vi "main_monitor_Rev_17x.vi"() -> ()   [LabVIEW 2012]
uses:
  <vilib>/measure/mamon.llb/Trigger Detection for 1 Channel.vi
  <vilib>/Analysis/3filter.llb/Butterworth Filter (DBL).vi
  <vilib>/measure/matone.llb/Extract Single Tone Information 1 Chan.vi
  <vilib>/measure/NI_MAPro.lvlib
  <vilib>/Analysis/NI_AALBase.lvlib
panel:
  out "# of bytes written":dbl
  out "String":string
  out "Array":dbl[](array[numeric])
  out "Delay":u32
  in  "SHIFT INPUT1 L SEL":bool
  in  "SHIFT INPUT2 R SEL":bool
  out "INPU1 shift sign":dbl
  out "INPUT2 shift sign":dbl
  out "Message":string
  out "Message 2":string
  out "Loop Count":i32
  out "Sent Command":string
  out "Shift INPUT2 R":dbl
  out "Shift INPUT1 L":dbl
  in  "Input buffer size 2":u32=16384
  out "Connected to Name":string
  out "Range Sel IN1 in":dbl format="%.2f"
  out "Range Sel IN2 in":dbl format="%.2f"
  out "Divider INPUT1 L":dbl
  out "Divider INPUT2 R":dbl
  out "Available COM ports":string[](array[string])
  out "Current time 2":timestamp
  out "#of sent bytes":dbl
  out "Lower Loc":dbl
  out "Upper Loc":dbl
  out "Running":bool
  out "Number of Samples":dbl
  out "Bytes at Port":u32
  out "Actual bytes read":u32
  in  "Input buffer size":u32=16384
  in  "baud rate":u32=1200000
  out "RESET USB":bool
  out "Connected to:":string
  in  "Select COM port":refnum<visa-resource-name>="COM3"
  in  "CNK":T1(tab)
  in  "Send New Configuration":bool
  in  "A/D settings":u16(ring)=1 items=["Set AD to 57 ksps", "Set AD to 3.56 ksps"]
  out "OL IN2":bool
  out "OL IN1":bool
  in  "Range select INPUT2":u16(ring) items=["+/- 0.6V", "+/- 18V", "+/- 110V", "+/- 450V"]
  in  "Range select INPUT1":u16(ring) items=["+/- 0.6V", "+/- 18V", "+/- 110V", "+/- 450V"]
  in  "AC /DC INPUT 2":bool
  in  "AC/DC INPUT 1":bool
  in  "View Select":T2(tab)
  out "Voltage":dynamicdata(graph)
  in  "Async send character":bool
  in  "Refresh Delay":dbl(knob)=46.47820132563531 scale=10.0..250.0
  out "Saved Value 2 IN1":dbl
  in  "Store Value 2 IN1":bool
  out "VDC INPUT1":dbl
  out "Number of data points":dbl
  out "Waveform Graph 2":dynamicdata(graph)
  out "Saved Value 1 IN1":dbl
  in  "Store Value 1 IN1":bool
  out "VDC INPUT2":dbl format="%#.6g"
  out "INPUT1 VAC Hz":dbl format="%#.6g"
  out "INPUT2 VAC Hz":dbl format="%#.6g"
  out "VMIN IN1":dbl format="%#.5g"
  out "VMAX CH1":dbl format="%#.5g"
  out "VMIN CH1":dbl format="%#.5g"
  out "VMAX IN1":dbl format="%#.5g"
  out "VRMS INPUT2":dbl format="%#.6g"
  out "VRMS INPUT1":dbl format="%#.6g"
  out "IN1 - IN2 V shift":dbl
  out "IN1/IN2 V gain":dbl
  in  "Store Value 1 IN2":bool
  out "Saved Value 1 IN2":dbl
  out "Saved Value 2 IN2":dbl
  in  "Store Value 2 IN2":bool
  in  "INPUT 2R Loc":dbl step=0.001
  in  "INPUT 1L Loc":dbl step=0.001
  in  "Zoom In Graph --->":dbl(slide)=0.573803 min=0.0 max=0.65 step=0.001 scale format="%#_1g"
  in  "Char to send":string="6"
  out "FFT":dynamicdata(graph)
  in  "Zoom In Graph ---> 2":dbl(slide)=1000.0 min=0.0 max=0.65 step=0.001 scale format="%#_1g"
  in  "Play Button":bool
  in  "Zoom In Graph ---> 3":dbl(slide)=0.573803 min=0.0 max=0.65 step=0.001 scale format="%#_1g"
  in  "Record single value":bool
  in  "Select path and filename":path
  in  "Continuous Rec Data CH0":bool
  out "Recorded data":waveform(dbl)[](graph)
  in  "Stop Playing":bool
  in  "Play Speed":i32(knob)=1000 scale=100.0..2000.0
  out "Reply 8":string
  out "Reply 7":string
  out "Reply 6":string
  out "Reply 5":string
  out "LB address 2":string
  out "HB address 2":string
  out "UB address 2":string
  out "MB address 2":string
  out "Data String CH0":string
  in  "Enable memory wright":bool
  out "Sign Address 2":string
  in  "Value of sign CH1":u8
  in  "Value of sign":u8
  out "Sign Address":string
  out "LB address":string
  out "HB address":string
  out "UB address":string
  out "MB address":string
  in  "WRITE INPUT1":bool
  out "LB data 2":u8
  out "HB data 2":u8
  out "UB data 2":u8
  out "MB  data 2":u8
  out "CH1 shift val HEX uV":u32 format="%x"
  out "CH1 Shift value uV":dbl format="%#_6f"
  out "LB data":u8
  out "HB data":u8
  out "UB data":u8
  out "MB data":u8
  out "CH0 shift val HEX uV":u32 format="%x"
  out "CH0 Shift value uV":dbl format="%#_6f"
  in  "WRITE INPUT2":bool
  in  "Enable cal":bool
  out "Reply 1":string
  out "Reply 2":string
  out "Reply 3":string
  out "Reply 4":string
  in  "Cal Voltage IN2":dbl
  out "Cal to Saved IN2":dbl
  in  "Cal Voltage IN1":dbl
  in  "PAUSE F1":bool
  in  "Continuous":bool=TRUE
  in  "STOP":bool
  in  "Single shot":bool
  in  "DC Filter":bool
  in  "Auto / Manual":bool=TRUE
  in  "MCU Reset":bool
  in  "View":u16(ring) items=["Both Inputs", "Input A", "Input B"]
  in  "Command":u16(ring)=1 items=["Read 256 bytes", "Read Both Channels", "Request Dividers", "Read Input 2 only", "Read Input 1 only", "Pause", "Single sample"]
  in  "Tab Control":T3(tab)
  in  "Filter Type":u16(ring) items=["Lowpass", "Highpass", "Bandpass", "Bandstop"]
  in  "Order":dbl=2.0
  in  "Low Cut Off":dbl=20000000.0
  in  "High Cutt Off":dbl=1.0
  in  "Sampling Frequency":dbl=100000000.0
  in  "Ymin":dbl=-2.0
  in  "Ymax":dbl=2.0
  out "OSCOPE":waveform(dbl)(graph)
  in  "DC SHIFT  1/10":dbl=-1.74
  in  "DC SHIFT  1/1":dbl=-1.77
  in  "Cal Gain 1/1":dbl=1.939
  in  "Cal Gain 1/10":dbl=10.555
  in  "Min y":dbl=-110.0
  in  "Max  y":dbl=-10.0
  in  "Min x":dbl
  in  "Max x":dbl=100000.0
  out "Graph 2":cluster{"f0":dbl, "df":dbl, "magnitude":dbl[]}(graph)
  in  "Minimum":dbl=-5.0
  in  "Maximum":dbl=5.0
  out "Waveform Graph 3":dbl[](graph)
  in  "Y min":dbl=-5.0
  in  "Y max":dbl=5.0
  out "Waveform Chart":dbl(graph)
  out "XY Graph":cluster{"Y":dbl[], "Y":dbl[]}[](graph)
  in  "Input Voltage Dividor":bool
  in  "Trigger Level":dbl step=0.01
  out "Frequency Hz":dbl
  out "Min":dbl
  out "Max":dbl
  in  "EXIT 2":bool
  in  "PAUSE 2":bool
  in  "Zoom In Wave --->":dbl(slide)=0.012286 min=0.0 max=0.012286 step=0.001 scale format="%#_1g"
  in  "Text Ring":u16(ring) items=["Falling Edge", "Rising Edge"]
  out "VDC":dbl
  out "Trigger Loc Index":dbl
  in  "Delay (ms)":dbl(knob)=106.62422249232296 scale=89.0..2000.0
  in  "AC/DC":bool
  out "x10":bool
  out "x1":bool
  in  "Ring":u16(ring) items=["Capacitance Numeric", "Capacitance Graph", "Resistance test graph", "Resistance test  270k", "Resistance test 27k", "Resistance test 2.7k", "Resistance test 270", "Resistance test 27"]
  in  "Apply current setting":bool
  in  "Tab Control 2":enum32{"Capacitance", "Resistance"}(tab)
  out "VCH1":dynamicdata(graph)
  out "Units":string
  out "Resistance Test":dynamicdata(graph)
  out "CH1 Vave":dbl
  out "Resistance":dbl
  in  "Exit":bool
  out "Apply Ind":bool
  in  "1. Apply Command":bool
  out "Frequency Hz 2":dbl
  in  "Period 2":u16=10 min=10 max=65000 step=1
  out "Period":string
  out "Waveform Graph":dynamicdata(graph)
  in  "% Duty Cycle":dbl=5.0 min=0.01 max=99.99 step=0.01
  out "Duty cycle":string
  in  "Stop Button":bool
  out "Number of bytes written":dbl
  out "T command Bytes sent":dbl
  in  "Erase All Data?":bool
  in  "Time Interval 0-9 sec":string="1"
  out "CH1 multiplier":dbl
  out "CH0 multiplier":dbl
  out "Data Read from memory HEX":string
  in  "Function Select":u16(ring) items=["Upload Data", "Erase Sector", "Download configuration", "Read memory location", "Record data", "Recod Dummy Data"]
  out "V data logger":dynamicdata(graph)
  in  "X-max 2":dbl(slide)=2048.0 scale=0.0..2048.0
  in  "Apply":bool
  out "Memory Responce":string
  out "Current time":timestamp
  in  "Voltage Range CH0":u16(ring) items=["+/- 0.6V", "+/- 18V", "+/- 110V", "+/- 450V"]
  in  "Voltage Range CH1":u16(ring) items=["+/- 0.6V", "+/-18V", "+/- 110V", "+/- 450V"]
  out "Divider CH0 Replied back":string
  out "Divider CH1 Replied back":string
  in  "Enter mem address in 5 decimal values. Example: 06142":string
  in  "STOP":bool
  in  "Send Configuration":bool
  in  "Range select INPUT2 2":u16(ring) items=["+/- 0.6V", "+/- 9V", "+/- 55V", "+/- 450V"]
  in  "Range select INPUT1 2":u16(ring) items=["+/- 0.6V", "+/- 9V", "+/- 55V", "+/- 450V"]
  in  "Memory Functions":u16(ring) items=["Upload Data", "Erase Sector", "Download configuration", "Read memory location", "Record data with datalogger", "Recod Dummy Data", "Erase calibration", "Get divider values and shift", "Reset", "CH0 set to 1/1", "CH0 set to 510k", "CH0 set to 80.6k", "CH0 set to 10k"]
  in  "Apply Memory Command":bool
  out "Reply":string
  in  "Stop Manual Range Select":bool=TRUE
  in  "Data Rate (u-sec)":string="1"
  in  "X-min":dbl
  in  "X-max":dbl=1000.0
  out "Number of Data Packs":dbl
  in  "minimum":dbl=-0.5
  in  "maximum":dbl=1.5
  in  "Stop Data Aquisition":bool
  out "Data Bytes":dbl
  out "Data Waveform":dynamicdata(graph)
  in  "Loop Delay":i32=1000
  # "1.2sec"
  # "L"
  # "R"
  # "i - Reply with board"
  # "'s' - collect and send 256 samples to PCUI"
  # "'v' erase calibration values"
  # "24 bit resolution"
  # "Cursor Navigation"
  # "24 bit resolution"
  # "INPUT 1 LEFT ch1"
  # "INPUT 2 RIGHT ch0"
  # "VDC"
  # "VDC"
  # "VAC"
  # "VAC"
  # "Hz"
  # "Hz"
  # "'W' - write MCP3911 registers"
  # "24 bit resolution"
  # "Select path and file name before recording the data."
  # "4 byte address"
  # "4 byte address"
  # "Decimal Value"
  # "Decimal Value"
  # "4"
  # "5"
  # "6"
  # "7"
  # "10 bit resolution"
  # "250Hz"
  # "22kHz"
  # "Component test results displayed on CH1"
  # "Values read back from memory on \"Upload Data\" operation"
  # "One data pack = 6144 bytes"
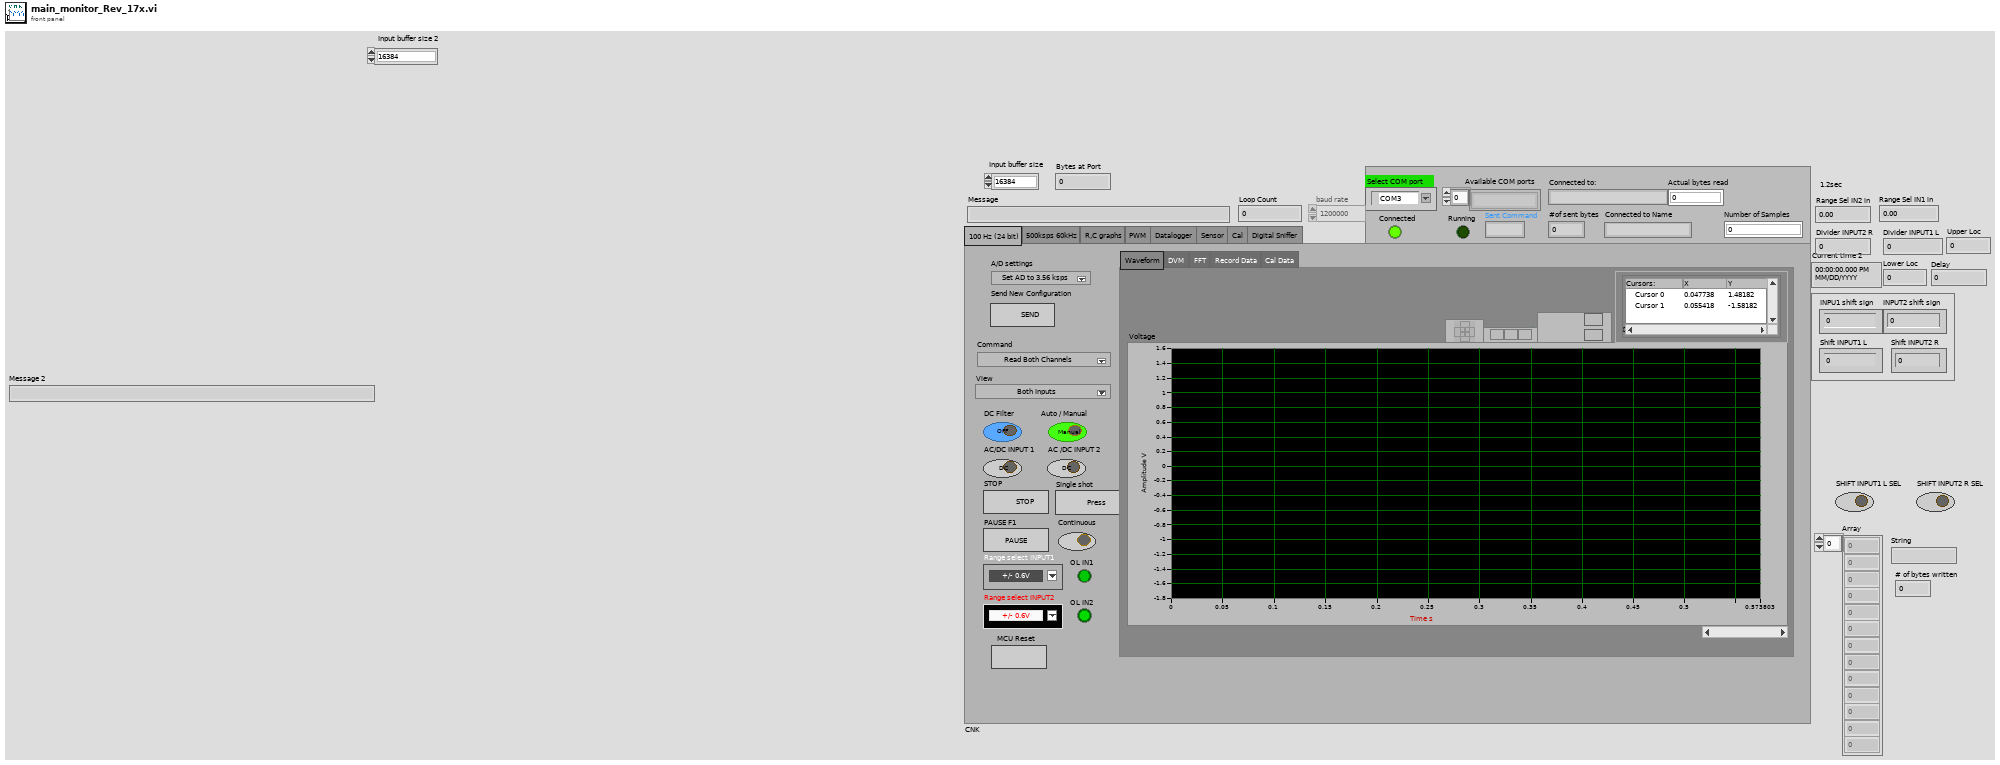
[diagram p1: front panel]
types:
  T1 = enum32{"100 Hz (24 bit)", "500ksps 60kHz", "R,C graphs", "PWM", "Datalogger", "Sensor", "Cal", "Digital Sniffer"}
  T2 = enum32{"Waveform", "DVM", "FFT", "Record Data", "Cal Data"}
  T3 = enum32{"Wave", "Spectrum", "sample number", "Chart", "XY Graph"}
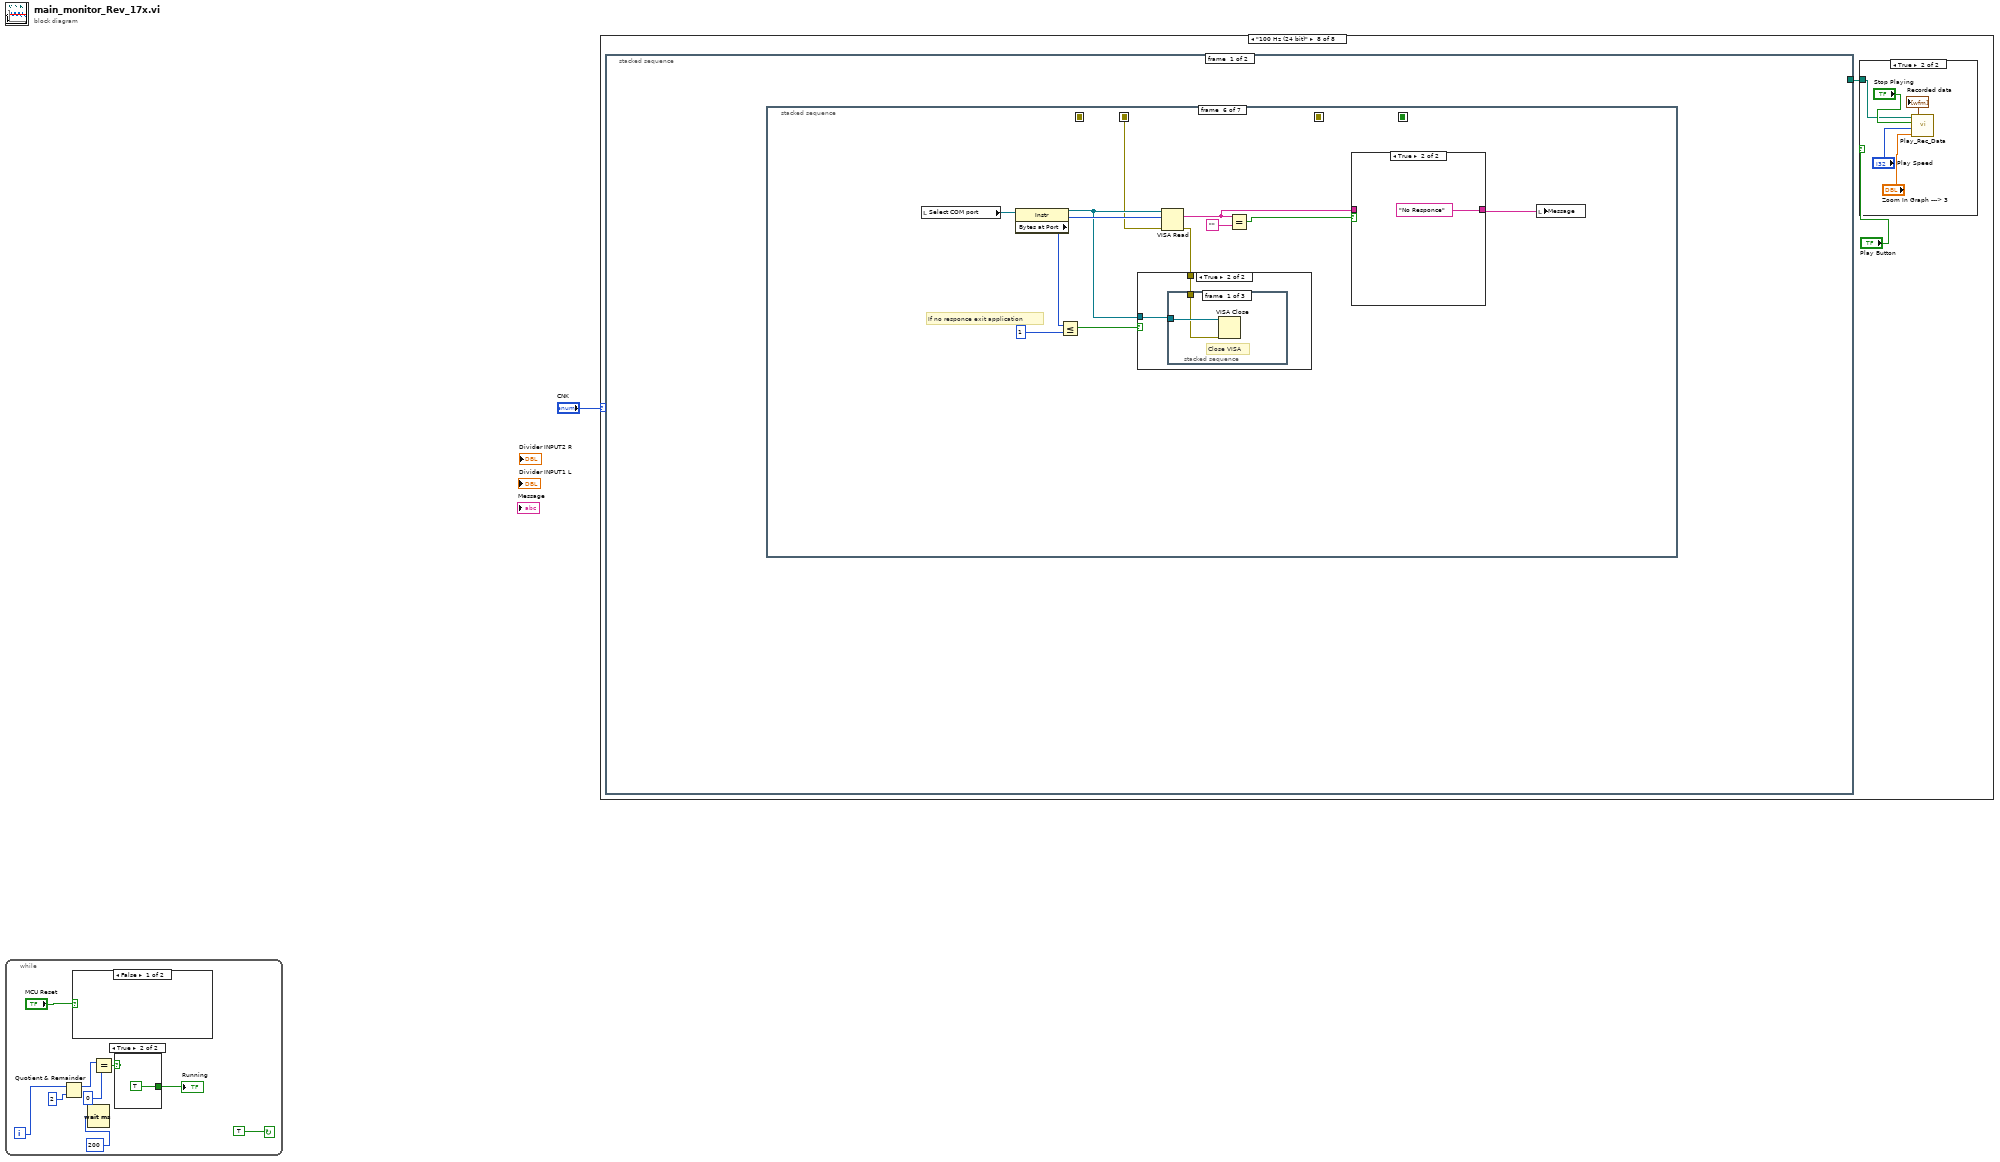
[diagram p0: block diagram]
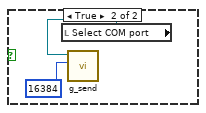
[diagram p2: hidden frame]
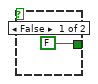
[diagram p3: hidden frame]
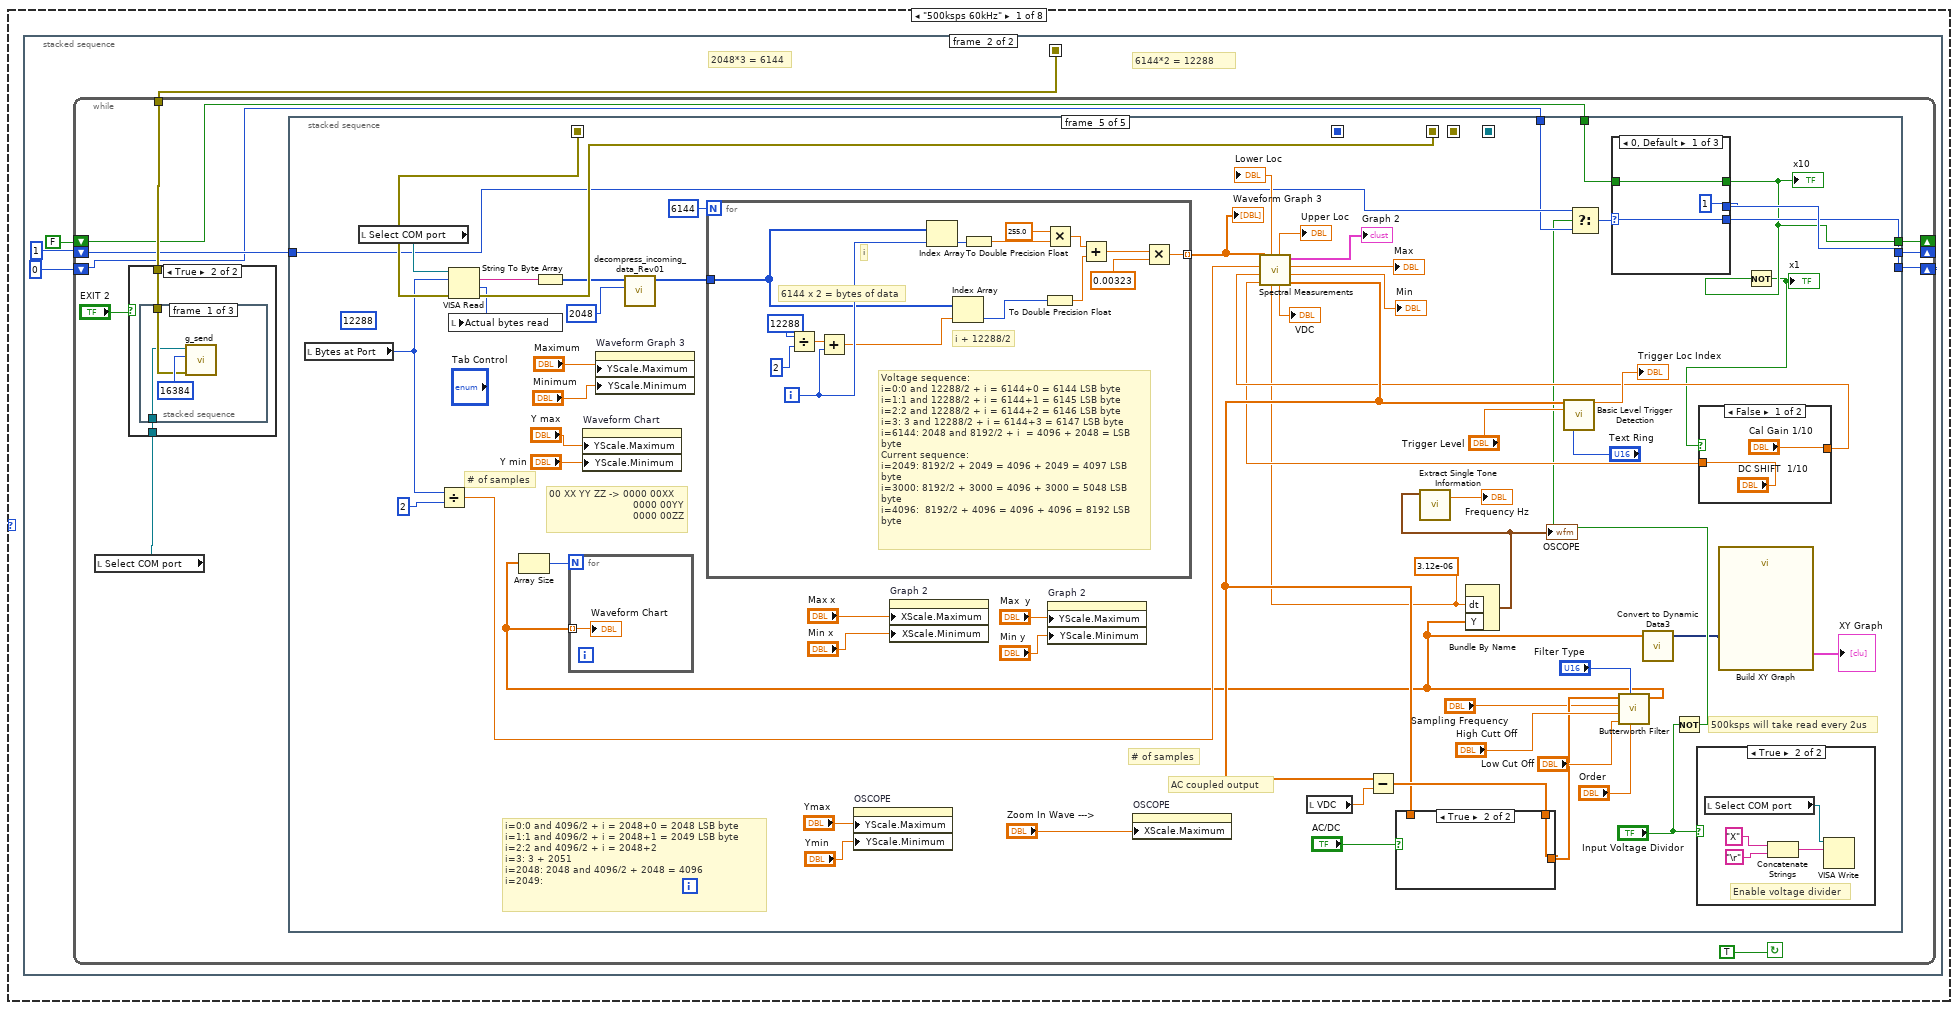
[diagram p4: hidden frame]
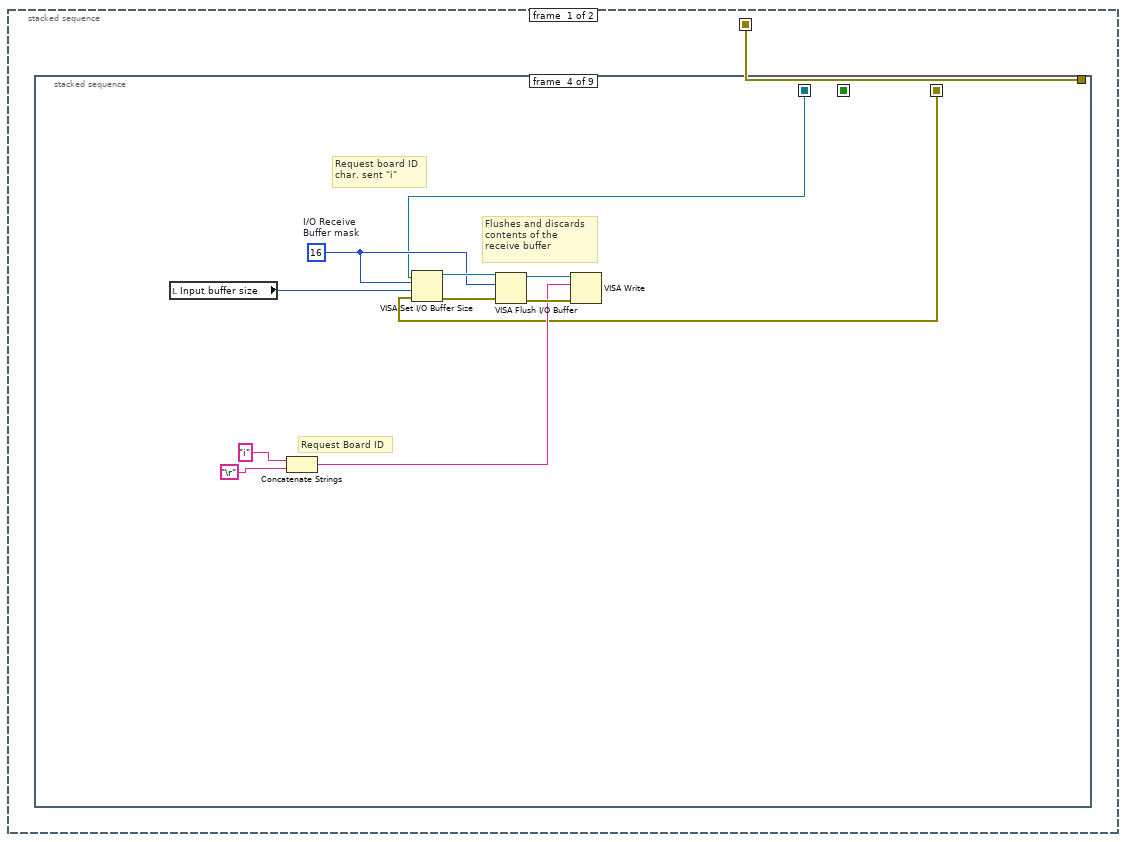
[diagram p5: hidden frame]
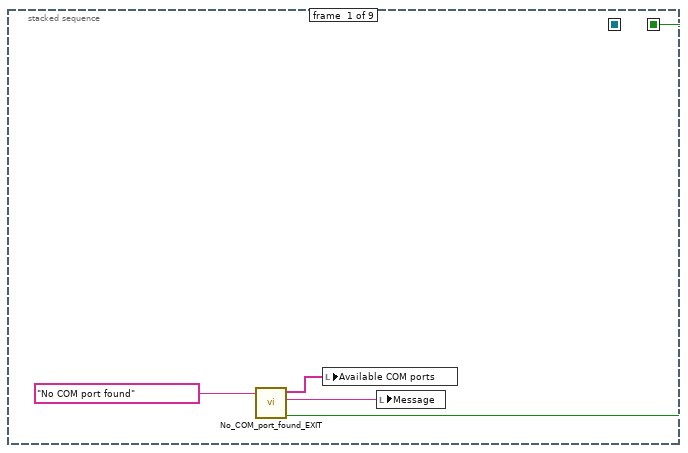
[diagram p6: hidden frame]
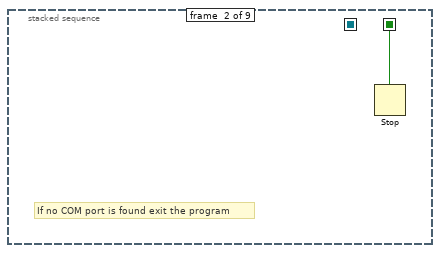
[diagram p7: hidden frame]
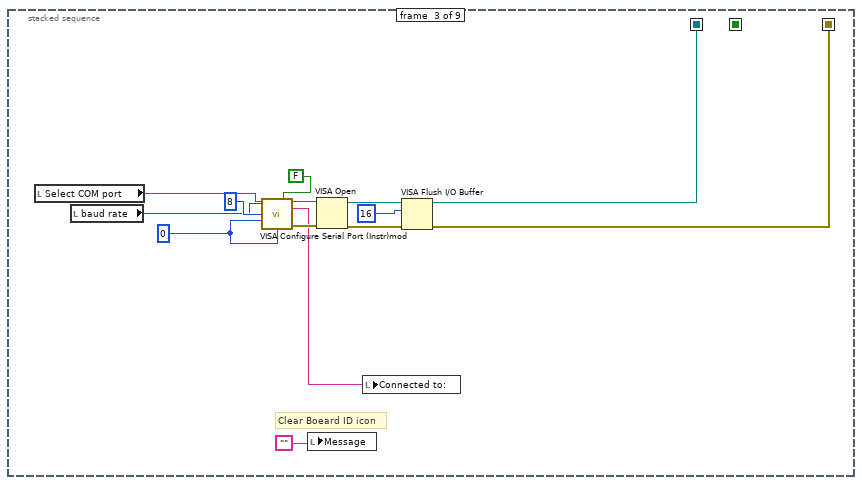
[diagram p8: hidden frame]
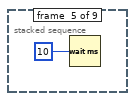
[diagram p9: hidden frame]
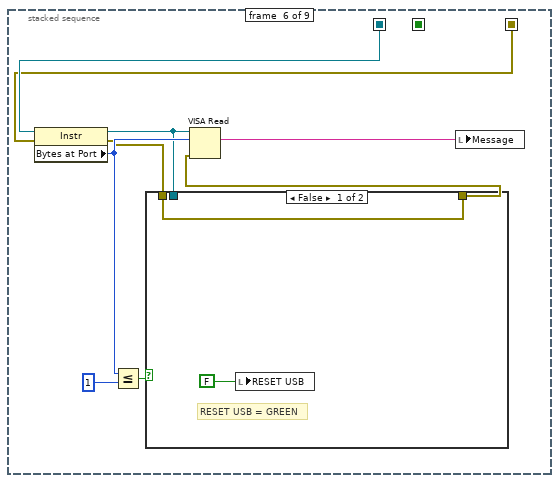
[diagram p10: hidden frame]
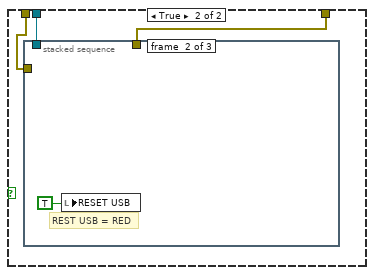
[diagram p11: hidden frame]
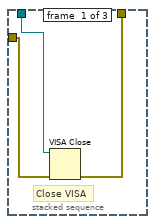
[diagram p12: hidden frame]
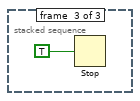
[diagram p13: hidden frame]
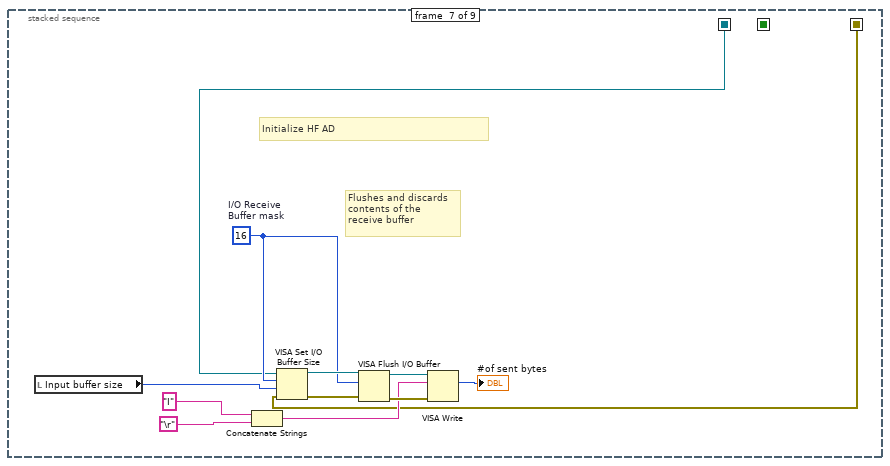
[diagram p14: hidden frame]
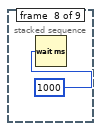
[diagram p15: hidden frame]
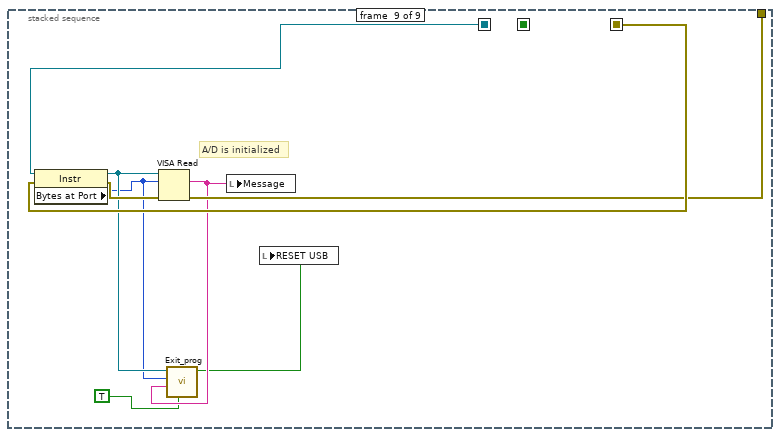
[diagram p16: hidden frame]
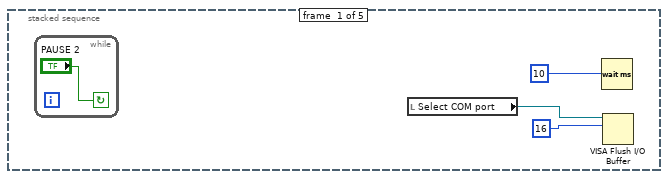
[diagram p17: hidden frame]
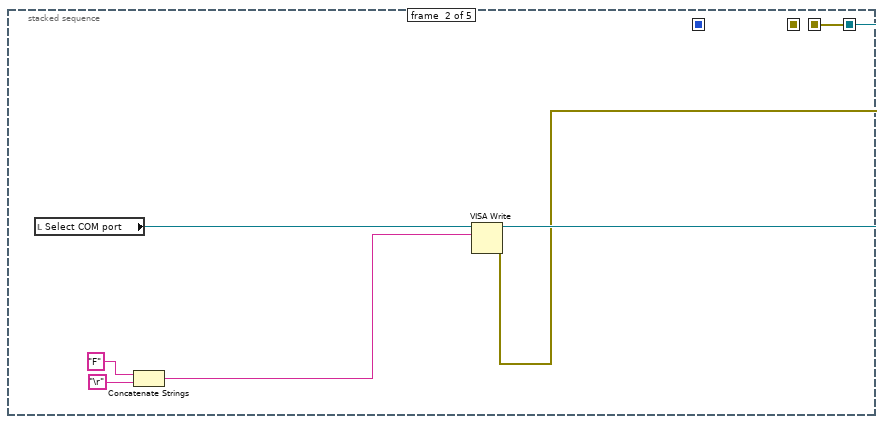
[diagram p18: hidden frame]
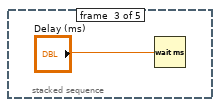
[diagram p19: hidden frame]
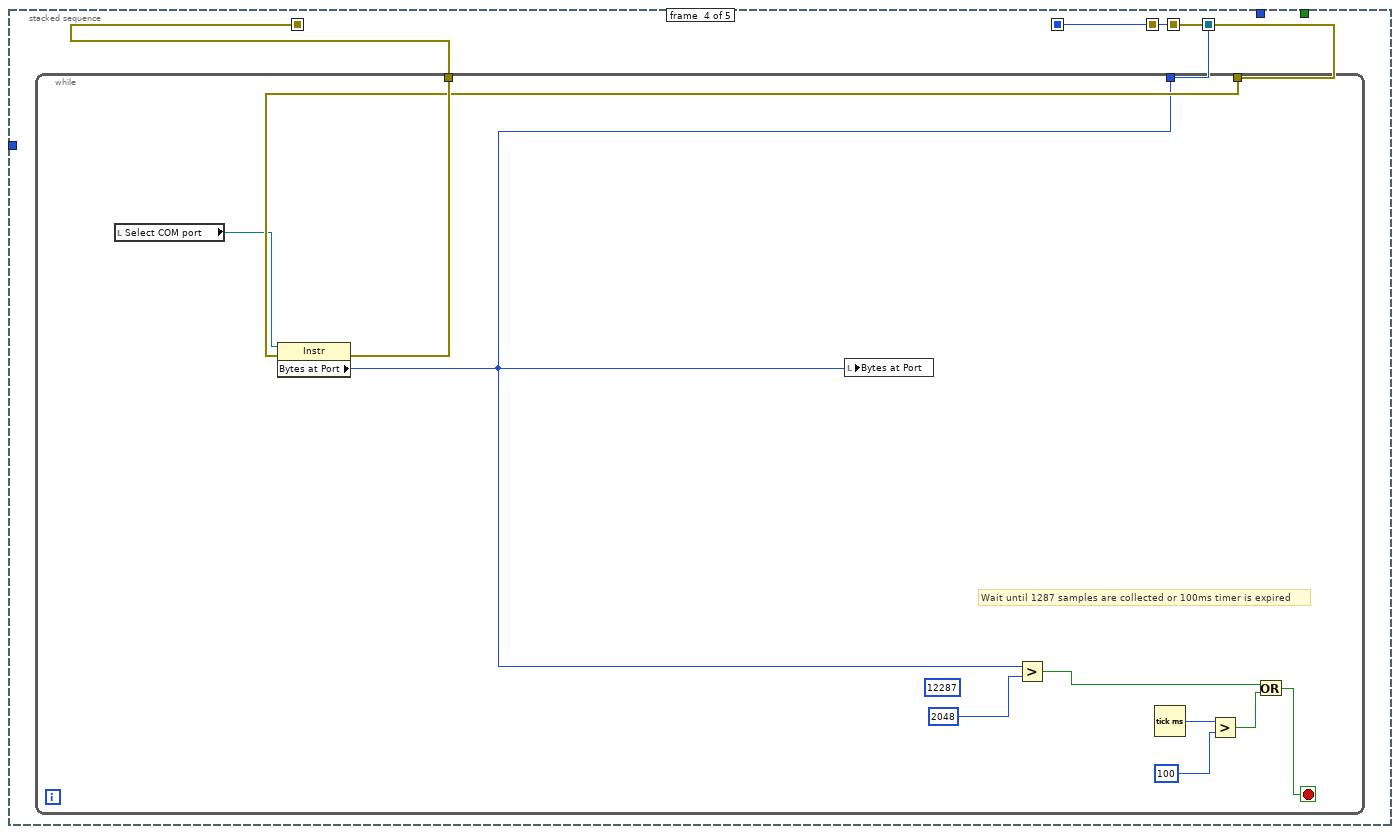
[diagram p20: hidden frame]
diagram:
  n1 = while {
    i -> [w6]
    stop <- TRUE continue-if-true
    n2 = Quotient & Remainder(x=w6, y=2) -> (x-y*floor(x/y)=w8:i32)  [unwired: 1 out]
    n3 = case shown="False" "MCU Reset" {
      frame False {
      }
      frame True {
        n4 = local read "Select COM port"() -> (w12:refnum<visa-resource-name>)
        n5 = call "g_send.vi"("Input buffer size"=16384, "USB Interface Name"=w12) -> ()  [unwired: 9 in, 1 out]
      }
    }
    n6 = Wait (ms)(milliseconds to wait=200) -> ()  [unwired: 1 out]
    n7 = Equal?(x=w8, y=0) -> (x = y?=w9:bool)
    n8 = case shown="True" w9 {
      tunnel: [FALSE TRUE] -> w5
      frame False {
      }
      frame True {
      }
    }
    "Running" <- w5
  }
  n9 = case shown="\"100 Hz (24 bit)\"" "CNK" {
    frame "500ksps 60kHz" {
      n10 = stacked-sequence {
        seq-local: [w15 _] -> [_ w88]
        frame #0 {
          n11 = stacked-sequence {
            seq-local: [_ _ w25 _ _ _ _ _ _] -> [_ _ _ w37 _ w49 w67 _ w85]
            seq-local: [_ _ w24 _ _ _ _ _ _] -> [_ _ _ w36 _ w50 w68 _ w86]
            seq-local: [w16 _ _ _ _ _ _ _ _] -> [_ w20 _ _ _ _ _ _ _]
            tunnel: [_ _ _ _ _ _ _ _ w82] -> w15
            frame #0 {
              n12 = call "No_COM_port_found_EXIT.vi"("Message In"="No COM port found") -> ("STOP"=w16:bool, "Message Out"=w18:string, "COM PORTS"=w17:string[])  [unwired: 6 in, 2 out]
              n13 = local write "Available COM ports"(w17) -> ()
              n14 = local write "Message"(w18) -> ()
            }
            frame #1 {
              # "If no COM port is found exit the program"
              n15 = Stop(stop? (T)=w20) -> ()
            }
            frame #2 {
              w33 = 0
              # "Clear Boeard ID icon"
              n16 = local read "Select COM port"() -> (w23:refnum<visa-resource-name>)
              n17 = local read "baud rate"() -> (w21:u32)
              n18 = call "VISA Configure Serial Port (Instr)mod.vi"("VISA resource name"=w23, "Enable Termination\nChar (T)"=FALSE, "baud rate (9600)"=w21, "data bits (8)"=8, "parity (0:none)"=w33, "flow control (0:none)"=w33) -> ("VISA resource name out"=w29:refnum<visa-resource-name>, "Name"=w22:string, "error out"=w30:errorcluster)  [unwired: 6 in, 1 out]
              n19 = local write "Message"("") -> ()
              n20 = VISA Open(error in (no error)=w30, VISA resource name=w29) -> (VISA resource name=w31:refnum<visa-resource-name>, error out=w32:errorcluster)  [unwired: 3 out]
              n21 = local write "Connected to:"(w22) -> ()
              n22 = VISA Flush I/O Buffer(VISA resource name=w31, mask (16)=u16 16 ("Maskieren (16)"), error in (no error)=w32) -> (VISA resource name out=w24:refnum<visa-resource-name>, error out=w25:errorcluster)
            }
            frame #3 {
              w41 = u16 16  # I/O Receive Buffer mask
              # "Request board ID\nchar. sent \"i\""
              # "Request Board ID"
              # "Flushes and discards \ncontents of the \nreceive buffer"
              n23 = local read "Input buffer size"() -> (w35:u32)
              n24 = Concatenate Strings("i", "\r") -> (w39:string)
              n25 = VISA Set I/O Buffer Size(VISA resource name=w36, mask (16)=w41, size (4096)=w35, error in (no error)=w37) -> (VISA resource name out=w43:refnum<visa-resource-name>, error out=w42:errorcluster)
              n26 = VISA Flush I/O Buffer(VISA resource name=w43, mask (16)=w41, error in (no error)=w42) -> (VISA resource name out=w45:refnum<visa-resource-name>, error out=w44:errorcluster)
              n27 = VISA Write(VISA resource name=w45, write buffer=w39, error in (no error)=w44) -> ()  [unwired: 3 out]
            }
            frame #4 {
              n28 = Wait (ms)(milliseconds to wait=10) -> ()  [unwired: 1 out]
            }
            frame #5 {
              n29 = property class="Instr"(reference=w50, error in=w49) -> (reference out=w51:refnum<visa-resource-name>, error out=w48:errorcluster, "Bytes at Port"=w53:u32)
              n30 = Less Or Equal?(x=w53, y=1) -> (x <= y?=w55:bool)
              n31 = case shown="False" w55 {
                tunnel: w48 -> [w57 w60]
                tunnel: [w57 w59] -> w54
                tunnel: w51 -> [_ w58]
                frame False {
                  # "RESET USB = GREEN"
                  n32 = local write "RESET USB"(FALSE) -> ()
                }
                frame True {
                  n33 = stacked-sequence {
                    tunnel: w60 -> [w63 _ _]
                    tunnel: [w62 _ _] -> w59
                    tunnel: w58 -> [w61 _ _]
                    frame #0 {
                      # "Close VISA"
                      n34 = VISA Close(VISA resource name=w61, error in (no error)=w63) -> (error out=w62:errorcluster)
                    }
                    frame #1 {
                      # "REST USB = RED"
                      n35 = local write "RESET USB"(TRUE) -> ()
                    }
                    frame #2 {
                      n36 = Stop(stop? (T)=TRUE ("Stop? (T)")) -> ()
                    }
                  }
                }
              }
              n37 = VISA Read(VISA resource name=w51, byte count=w53, error in (no error)=w54) -> (read buffer=w47:string)  [unwired: 3 out]
              n38 = local write "Message"(w47) -> ()
            }
            frame #6 {
              w73 = u16 16  # I/O Receive Buffer mask
              # "Initialize HF AD"
              # "Flushes and discards \ncontents of the \nreceive buffer"
              n39 = local read "Input buffer size"() -> (w66:u32)
              n40 = Concatenate Strings("I", "\r") -> (w69:string)
              n41 = VISA Set I/O Buffer Size(VISA resource name=w68, mask (16)=w73, size (4096)=w66, error in (no error)=w67) -> (VISA resource name out=w75:refnum<visa-resource-name>, error out=w74:errorcluster)
              n42 = VISA Flush I/O Buffer(VISA resource name=w75, mask (16)=w73, error in (no error)=w74) -> (VISA resource name out=w77:refnum<visa-resource-name>, error out=w76:errorcluster)
              n43 = VISA Write(VISA resource name=w77, write buffer=w69, error in (no error)=w76) -> (return count=→"#of sent bytes":u32)  [unwired: 2 out]
            }
            frame #7 {
              n44 = Wait (ms)(milliseconds to wait=1000) -> ()  [unwired: 1 out]
            }
            frame #8 {
              # "A/D is initialized"
              n45 = property class="Instr"(reference=w86, error in=w85) -> (reference out=w84:refnum<visa-resource-name>, error out=w87:errorcluster, "Bytes at Port"=w83:u32)
              n46 = VISA Read(VISA resource name=w84, byte count=w83, error in (no error)=w87) -> (read buffer=w81:string, error out=w82:errorcluster)  [unwired: 2 out]
              n47 = call "Exit_prog.vi"("EN/DIS"=TRUE, "InputStr"=w81, "Bytes to read"=w83, "USB Interface Name"=w84) -> ("RESET USB"=w80:bool)  [unwired: 5 in, 2 out]
              n48 = local write "Message"(w81) -> ()
              n49 = local write "RESET USB"(w80) -> ()
            }
          }
        }
        frame #1 {
          # "6144*2 = 12288"
          # "2048*3 = 6144"
          n50 = while {
            tunnel: w88 -> [w101]
            shift-right: [w97] -> _
            shift-left: FALSE ("Toggle") -> [w94]
            shift-right: [w96] -> _
            shift-left: 1 -> [w93]
            shift-right: [w95] -> _
            shift-left: 0 -> [w92]
            stop <- TRUE ("RUN") continue-if-true
            n51 = local read "Select COM port"() -> (w100:refnum<visa-resource-name>)
            n52 = case shown="True" "EXIT 2" {
              tunnel: w101 -> [_ w227]
              tunnel: w100 -> [_ w226]
              frame False {
              }
              frame True {
                n53 = stacked-sequence {
                  tunnel: w227 -> [w229 _ _]
                  tunnel: w226 -> [w228 w231 _]
                  frame #0 {
                    n54 = call "g_send.vi"("error in (no error)"=w229, "Input buffer size"=16384, "USB Interface Name"=w228) -> ()  [unwired: 8 in, 1 out]
                  }
                  frame #1 {
                    n55 = VISA Close(VISA resource name=w231) -> ()  [unwired: 1 in, 1 out]
                  }
                  frame #2 {
                    n56 = Stop(stop? (T)=TRUE ("Stop? (T)")) -> ()
                  }
                }
              }
            }
            n57 = stacked-sequence {
              seq-local: [_ w108 _ _ _] -> [_ _ _ _ _]
              seq-local: [_ w107 _ _ _] -> [_ _ _ w114 _]
              seq-local: [_ _ _ w115 _] -> [_ _ _ _ w186]
              seq-local: [_ _ _ _ w187] -> [_ _ _ _ _]
              seq-local: [_ _ _ w113 _] -> [_ _ _ _ _]
              tunnel: [_ _ _ _ w147] -> w97
              tunnel: [_ _ _ _ w153] -> w96
              tunnel: [_ _ _ _ w152] -> w95
              tunnel: w94 -> [_ _ _ _ w151]
              tunnel: w93 -> [_ _ _ _ w150]
              tunnel: w92 -> [_ _ _ _ w149]
              frame #0 {
                n58 = while {
                  stop <- "PAUSE 2" continue-if-true
                }
                n59 = local read "Select COM port"() -> (w102:refnum<visa-resource-name>)
                n60 = Wait (ms)(milliseconds to wait=10) -> ()  [unwired: 1 out]
                n61 = VISA Flush I/O Buffer(VISA resource name=w102, mask (16)=u16 16 ("Maskieren (16)")) -> ()  [unwired: 1 in, 2 out]
              }
              frame #1 {
                n62 = local read "Select COM port"() -> (w106:refnum<visa-resource-name>)
                n63 = Concatenate Strings("F", "\r") -> (w110:string)
                n64 = VISA Write(VISA resource name=w106, write buffer=w110) -> (VISA resource name out=w108:refnum<visa-resource-name>, error out=w107:errorcluster)  [unwired: 1 in, 1 out]
              }
              frame #2 {
                n65 = Wait (ms)(milliseconds to wait="Delay (ms)") -> ()  [unwired: 1 out]
              }
              frame #3 {
                n66 = while {
                  tunnel: [w125] -> w115
                  tunnel: w114 -> [w124]
                  tunnel: [w123] -> w113
                  stop <- w122 stop-if-true
                  (unwired) 12287
                  # "Wait until 1287 samples are collected or 100ms timer is expired"
                  n67 = local read "Select COM port"() -> (w116:refnum<visa-resource-name>)
                  n68 = property class="Instr"(reference=w116, error in=w124) -> (error out=w125:errorcluster, "Bytes at Port"=w123:u32)  [unwired: 1 out]
                  n69 = local write "Bytes at Port"(w123) -> ()
                  n70 = Greater?(x=w123, y=2048) -> (0:w121:bool)
                  n71 = Tick Count (ms)() -> (millisecond timer value=w118:u32)
                  n72 = Greater?(x=w118, y=100) -> (0:w120:bool)
                  n73 = Or(x=w121, y=w120) -> (x .or. y?=w122:bool)
                }
              }
              frame #4 {
                (unwired) 12288
                w130 = 3.12e-06
                # "00 XX YY ZZ -> 0000 00XX\n                            0000 00YY\n                            0000 00ZZ"
                # "# of samples"
                # "AC coupled output"
                # "500ksps will take read every 2us"
                # "# of samples"
                # "i=0:0 and 4096/2 + i = 2048+0 = 2048 LSB byte\ni=1:1 and 4096/2 + i = 2048+1 = 2049 LSB byte\ni=2:2 and 4096/2 + i = 2048+2\ni=3: 3 + 2051\ni=2048: 2048 and 4096/2 + 2048 = 4096\ni=2049:"
                n74 = local read "Bytes at Port"() -> (w172:u32)
                n75 = local read "Select COM port"() -> (w177:refnum<visa-resource-name>)
                n76 = Divide(x=w172, y=2) -> (x/y=w163:dbl)
                n77 = VISA Read(VISA resource name=w177, byte count=w172, error in (no error)=w186) -> (read buffer=w185:string, return count=w176:u32, error out=w187:errorcluster)  [unwired: 1 out]
                n78 = local write "Actual bytes read"(w176) -> ()
                n79 = String To Byte Array(string=w185) -> (unsigned byte array=w173:u8[])
                n80 = property on="Waveform Chart" class="WFChart (strict)"("YScale.Maximum"="Y max", "YScale.Minimum"="Y min") -> ()  [unwired: 2 in, 2 out]
                n81 = property on="Waveform Graph 3" class="WFGraph (strict)"("YScale.Maximum"="Maximum", "YScale.Minimum"="Minimum") -> ()  [unwired: 2 in, 2 out]
                n82 = call "decompress_incoming_data_Rev01.vi"("N"=2048, "Input Data"=w173) -> ("Combined output binary values"=w167:u8[])  [unwired: 7 in]
                n83 = for {
                  N: 6144 -> [_]
                  tunnel: w167 -> [w212]
                  tunnel: [w219] -> w138 mode=indexing
                  i -> [w216]
                  # "Voltage sequence:\ni=0:0 and 12288/2 + i = 6144+0 = 6144 LSB byte \ni=1:1 and 12288/2 + i = 6144+1 = 6145 LSB byte\ni=2:2 and 12288/2 + i = 6144+2 = 6146 LSB byte\ni=3: 3 and 12288/2 + i = 6144+3 = 6147 LSB byte\ni=6144: 2048 and 8192/2 + i  = 4096 + 2048 = LSB byte\nCurrent sequence:\ni=2049: 8192/2 + 2049 = 4096 + 2049 = 4097 LSB byte\ni=3000: 8192/2 + 3000 = 4096 + 3000 = 5048 LSB byte\ni=4096:  8192/2 + 4096 = 4096 + 4096 = 8192 LSB byte"
                  # "i + 12288/2"
                  # "i"
                  # "6144 x 2 = bytes of data"
                  n84 = Divide(x=12288, y=2) -> (x/y=w217:dbl)
                  n85 = Add(x=w217, y=w216) -> (x+y=w215:dbl)
                  n86 = Index Array(array=w212, index=w216) -> (element=w213:u8)
                  n87 = Index Array(array=w212, index=w215) -> (element=w214:u8)
                  n88 = To Double Precision Float(number=w213) -> (double precision float=w224:dbl)
                  n89 = Multiply(x=255.0, y=w224) -> (x*y=w223:dbl)
                  n90 = To Double Precision Float(number=w214) -> (double precision float=w222:dbl)
                  n91 = Add(x=w223, y=w222) -> (x+y=w221:dbl)
                  n92 = Multiply(x=w221, y=0.00323) -> (x*y=w219:dbl)
                }
                "Waveform Graph 3" <- w138
                n93 = property on="OSCOPE" class="WFGraph (strict)"("YScale.Maximum"="Ymax", "YScale.Minimum"="Ymin") -> ()  [unwired: 2 in, 2 out]
                n94 = property on="Graph 2" class="WFGraph (strict)"("XScale.Maximum"="Max x", "XScale.Minimum"="Min x") -> ()  [unwired: 2 in, 2 out]
                n95 = property on="Graph 2" class="WFGraph (strict)"("YScale.Maximum"="Max  y", "YScale.Minimum"="Min y") -> ()  [unwired: 2 in, 2 out]
                n96 = property on="OSCOPE" class="WFGraph (strict)"("XScale.Maximum"="Zoom In Wave --->") -> ()  [unwired: 2 in, 2 out]
                n97 = local read "VDC"() -> (w179:dbl)
                n98 = Not(x="Input Voltage Dividor") -> (.not. x?=w144:bool)
                n99 = Select(t=w150, s=w144, f=w149) -> (s? t:f=w148:i32)
                n100 = case shown="0, Default" w148 {
                  selector: w148 -> [w189 w192 _]
                  tunnel: [w190 w191 w194] -> w147
                  tunnel: w151 -> [w190 w191 w195]
                  tunnel: [w189 2 0] -> w152
                  tunnel: [1 w192 1] -> w153
                  frame 0, Default {
                  }
                  frame 1 {
                  }
                  frame 2 {
                    n101 = Not(x=w195) -> (.not. x?=w196:bool)
                    n102 = Select(t=w196, s=TRUE ("Toggle"), f=w195) -> (s? t:f=w194:bool)
                  }
                }
                "x10" <- w147
                n103 = case shown="True" "Input Voltage Dividor" {
                  frame False {
                  }
                  frame True {
                    # "Enable voltage divider"
                    n104 = local read "Select COM port"() -> (w207:refnum<visa-resource-name>)
                    n105 = Concatenate Strings("X", "\r") -> (w208:string)
                    n106 = VISA Write(VISA resource name=w207, write buffer=w208) -> ()  [unwired: 1 in, 3 out]
                  }
                }
                n107 = Not(x=w147) -> (.not. x?=w143:bool)
                "x1" <- w143
                n108 = case shown="False" w143 {
                  tunnel: ["Cal Gain 1/10" "Cal Gain 1/1"] -> w154
                  tunnel: ["DC SHIFT  1/10" "DC SHIFT  1/1"] -> w146
                  frame False {
                  }
                  frame True {
                  }
                }
                n109 = call "Spectral Measurements.vi"("dt"=w130, "DC SHIFT"=w146, "Voltage Divider IN"=w154, "Number of samples"=w163, "Array In"=w138) -> ("Array Out"=w162:dbl[], "Min"=→"Min":dbl, "Max"=→"Max":dbl, "Graph 2"=→"Graph 2":cluster{"f0":dbl, "df":dbl, "magnitude":dbl[]}, "VDC"=→"VDC":dbl, "Upper Loc"=→"Upper Loc":dbl, "Lower Loc"=→"Lower Loc":dbl)
                n110 = Subtract(x=w162, y=w179) -> (x-y=w169:dbl[])
                n111 = case shown="True" "AC/DC" {
                  tunnel: [w205 w206] -> w137
                  tunnel: w169 -> [_ w206]
                  tunnel: w162 -> [w205 _]
                  frame False {
                  }
                  frame True {
                  }
                }
                n112 = call-poly <vilib>:"Basic Level Trigger Detection.vi"("signal in"=w162, "level"="Trigger Level", "trigger slope"="Text Ring") -> ("trigger location"=→"Trigger Loc Index":dbl)  [unwired: 10 in, 2 out]
                n113 = call-poly <vilib>:"Butterworth Filter.vi"("order"="Order", "filter type"="Filter Type", "low cutoff freq: fl"="Low Cut Off", "high cutoff freq: fh"="High Cutt Off", "sampling freq: fs"="Sampling Frequency", "X"=w137) -> ("Filtered X"=w127:dbl[])  [unwired: 2 in, 1 out]
                n114 = Array Size(array=w127) -> (size(s)=w168:i32)
                n115 = for {
                  N: w168 -> [_]
                  tunnel: w127 -> [w204] mode=indexing
                  "Waveform Chart" <- w204
                }
                n116 = Bundle By Name("dt"=w130, "Y"=w127) -> (w136:waveform(dbl))  [unwired: 1 in]
                "OSCOPE" <- w136
                n117 = call-poly <vilib>:"Extract Single Tone Information.vi"("time signal in"=w136) -> ("detected frequency"=→"Frequency Hz":dbl)  [unwired: 5 in, 5 out]
                n118 = call "Convert to Dynamic Data3"("Array"=w127) -> ("Dynamic Data Type"=w126:dynamicdata)  [unwired: 3 in]
                n119 = call "Build XY Graph"("Y Input"=w126) -> ("XY Graph"=→"XY Graph":cluster{"Y":dbl[], "Y":dbl[]}[])  [unwired: 4 in, 6 out]
              }
            }
          }
        }
      }
    }
    frame "PWM" {
      n120 = stacked-sequence {
        seq-local: [w236 _ _] -> [_ w249 w285]
        frame #0 {
          w238 = 0
          # "CONNECT"
          # "Initialize serial interface"
          n121 = local read "Select COM port"() -> (w235:refnum<visa-resource-name>)
          n122 = local read "baud rate"() -> (w234:u32)
          n123 = call "VISA Configure Serial Port (Instr)mod.vi"("VISA resource name"=w235, "Enable Termination\nChar (T)"=FALSE, "baud rate (9600)"=w234, "data bits (8)"=8, "parity (0:none)"=w238, "flow control (0:none)"=w238) -> ("VISA resource name out"=w242:refnum<visa-resource-name>, "Name"=w233:string, "error out"=w241:errorcluster)  [unwired: 6 in, 1 out]
          n124 = VISA Open(error in (no error)=w241, VISA resource name=w242) -> (VISA resource name=w240:refnum<visa-resource-name>, error out=w239:errorcluster)  [unwired: 3 out]
          n125 = local write "Connected to:"(w233) -> ()
          n126 = VISA Flush I/O Buffer(VISA resource name=w240, mask (16)=u16 16 ("Maskieren (16)"), error in (no error)=w239) -> (error out=w236:errorcluster)  [unwired: 1 out]
        }
        frame #1 {
          n127 = flat-sequence {
            tunnel: w249 -> [w256]
            tunnel: [w255] -> w247
            tunnel: [w254] -> w245
            tunnel: [w264] -> w248
            tunnel: w247 -> [w264]
            tunnel: [w263] -> w246
            tunnel: w245 -> [w263]
            tunnel: w248 -> [w268]
            tunnel: w246 -> [w267]
            frame #0 {
              w258 = u16 16  # I/O Receive Buffer mask
              # "Clear Message window"
              # "Request board ID\nchar. sent \"i\""
              # "Request Board ID"
              # "Flushes and discards \ncontents of the \nreceive buffer"
              n128 = Concatenate Strings("i", "\r") -> (w257:string)
              n129 = local read "Select COM port"() -> (w250:refnum<visa-resource-name>)
              n130 = VISA Set I/O Buffer Size(VISA resource name=w250, mask (16)=w258, error in (no error)=w256) -> (VISA resource name out=w260:refnum<visa-resource-name>, error out=w259:errorcluster)  [unwired: 1 in]
              n131 = local write "Message"("") -> ()
              n132 = VISA Flush I/O Buffer(VISA resource name=w260, mask (16)=w258, error in (no error)=w259) -> (VISA resource name out=w262:refnum<visa-resource-name>, error out=w261:errorcluster)
              n133 = VISA Write(VISA resource name=w262, write buffer=w257, error in (no error)=w261) -> (VISA resource name out=w255:refnum<visa-resource-name>, error out=w254:errorcluster)  [unwired: 1 out]
            }
            frame #1 {
              n134 = Wait (ms)(milliseconds to wait=400) -> ()  [unwired: 1 out]
            }
            frame #2 {
              # "Receive board ID"
              n135 = property class="Instr"(reference=w268, error in=w267) -> (reference out=w271:refnum<visa-resource-name>, error out=w270:errorcluster, "Bytes at Port"=w273:u32)
              n136 = Less Or Equal?(x=w273, y=1) -> (x <= y?=w274:bool)
              n137 = case shown="True" w274 {
                tunnel: w271 -> [_ w279]
                tunnel: w270 -> [w275 w278]
                tunnel: [w275 w277] -> w269
                frame False {
                  # "RESET USB = GREEN"
                  n138 = local write "RESET USB"(FALSE) -> ()
                }
                frame True {
                  n139 = stacked-sequence {
                    tunnel: w279 -> [w282 _ _]
                    tunnel: w278 -> [w281 _ _]
                    tunnel: [w280 _ _] -> w277
                    frame #0 {
                      # "Close VISA"
                      n140 = VISA Close(VISA resource name=w282, error in (no error)=w281) -> (error out=w280:errorcluster)
                    }
                    frame #1 {
                      # "REST USB = RED"
                      n141 = local write "RESET USB"(TRUE) -> ()
                    }
                    frame #2 {
                      n142 = Stop(stop? (T)=TRUE ("Stop? (T)")) -> ()
                    }
                  }
                }
              }
              n143 = VISA Read(VISA resource name=w271, byte count=w273, error in (no error)=w269) -> (read buffer=w266:string)  [unwired: 3 out]
              n144 = local write "Message"(w266) -> ()
            }
          }
        }
        frame #2 {
          # "The main wlile() loop"
          n145 = stacked-sequence {
            seq-local: [w286 _ _ _ _ _ _ _ _] -> [_ w298 _ _ _ _ _ _ _]
            seq-local: [_ _ _ _ w314 _ _ _ _] -> [_ _ _ _ _ _ w400 _ _]
            seq-local: [_ _ _ _ _ w361 _ _ _] -> [_ _ _ _ _ _ w401 _ _]
            seq-local: [_ _ _ _ "Period 2" _ _ _ _] -> [_ _ _ _ _ w360 _ _ _]
            seq-local: [_ _ _ _ w310 _ _ _ _] -> [_ _ _ _ _ w355 _ _ _]
            tunnel: w285 -> [_ w299 _ _ _ _ w404 _ _]
            frame #0 {
              n146 = while {
                tunnel: [w288] -> w286
                stop <- "1. Apply Command" stop-if-true
                # "Stack 2 char"
                n147 = Wait (ms)(milliseconds to wait=100) -> ()  [unwired: 1 out]
                n148 = property on="Apply Ind" class="Bool (strict)"("Blinking"=FALSE) -> ()  [unwired: 2 in, 2 out]
                n149 = Concatenate Strings("1", "\r") -> (w288:string)
                "Apply Ind" <- TRUE
              }
            }
            frame #1 {
              w300 = u16 16  # I/O Receive Buffer mask
              # "Write command"
              # "Previously selected command is sent to the FB"
              # "Flushes and discards \ncontents of the \nreceive buffer"
              n150 = local read "Input buffer size"() -> (w295:u32)
              n151 = local read "Select COM port"() -> (w294:refnum<visa-resource-name>)
              n152 = local write "Apply Ind"(FALSE) -> ()
              n153 = VISA Set I/O Buffer Size(VISA resource name=w294, mask (16)=w300, size (4096)=w295, error in (no error)=w299) -> (VISA resource name out=w302:refnum<visa-resource-name>, error out=w301:errorcluster)
              n154 = VISA Flush I/O Buffer(VISA resource name=w302, mask (16)=w300, error in (no error)=w301) -> (VISA resource name out=w304:refnum<visa-resource-name>, error out=w303:errorcluster)
              n155 = VISA Write(VISA resource name=w304, write buffer=w298, error in (no error)=w303) -> (return count=→"Number of bytes written":u32)  [unwired: 2 out]
            }
            frame #2 {
              n156 = Wait (ms)(milliseconds to wait=20) -> ()  [unwired: 1 out]
            }
            frame #3 {
              n157 = local read "Select COM port"() -> (w306:refnum<visa-resource-name>)
              n158 = property class="Instr"(reference=w306) -> (reference out=w308:refnum<visa-resource-name>, "Bytes at Port"=w307:u32)  [unwired: 1 in, 1 out]
              n159 = VISA Read(VISA resource name=w308, byte count=w307) -> (read buffer=w309:string)  [unwired: 1 in, 3 out]
              n160 = local write "Message"(w309) -> ()
            }
            frame #4 {
              n161 = Less?(x="Period 2", y=10000) -> (x < y?=w315:bool)
              n162 = case shown="False" w315 {
                tunnel: [w317 w323] -> w314
                tunnel: "Period 2" -> [w318 w320]
                frame False {
                  n163 = Number To Decimal String(number=w318, width (-)=5) -> (decimal integer string=w317:string)
                }
                frame True {
                  n164 = Less?(x=w320, y=1000) -> (x < y?=w321:bool)
                  n165 = case shown="True" w321 {
                    tunnel: [w324 w330] -> w323
                    tunnel: w320 -> [w326 w329]
                    frame False {
                      # "greater then 1000"
                      n166 = Number To Decimal String(number=w326, width (-)=4) -> (decimal integer string=w327:string)
                      n167 = Concatenate Strings("0", w327) -> (w324:string)
                    }
                    frame True {
                      # "999"
                      n168 = Less?(x=w329, y=100) -> (x < y?=w332:bool)
                      n169 = case shown="True" w332 {
                        tunnel: [w333 w338] -> w330
                        tunnel: w329 -> [w336 w339]
                        frame False {
                          w334 = "0"
                          # "100 - 999"
                          # ">=100 <1000"
                          n170 = Number To Decimal String(number=w336, width (-)=3) -> (decimal integer string=w335:string)
                          n171 = Concatenate Strings(w334, w334, w335) -> (w333:string)
                        }
                        frame True {
                          n172 = Less?(x=w339, y=10) -> (x < y?=w341:bool)
                          n173 = case shown="True" w341 {
                            tunnel: w339 -> [w344 w348]
                            tunnel: [w342 w349] -> w338
                            frame False {
                              w343 = "0"
                              # "10 - 99"
                              # ">=10 but <100"
                              # "<100"
                              n174 = Number To Decimal String(number=w344, width (-)=2) -> (decimal integer string=w345:string)
                              n175 = Concatenate Strings(w343, w343, w343, w345) -> (w342:string)
                            }
                            frame True {
                              w347 = "0"
                              # "0-9"
                              # "<10"
                              n176 = Number To Decimal String(number=w348, width (-)=1) -> (decimal integer string=w350:string)
                              n177 = Concatenate Strings(w347, w347, w347, w347, w350) -> (w349:string)
                            }
                          }
                        }
                      }
                    }
                  }
                }
              }
              "Period" <- w314
              n178 = To Double Precision Float(number="Period 2") -> (double precision float=w311:dbl)
              n179 = Divide(x=14745000.0, y=w311) -> (x/y=w310:dbl)
              "Frequency Hz 2" <- w310
            }
            frame #5 {
              n180 = To Double Precision Float(number=w360) -> (double precision float=w358:dbl)
              n181 = Divide(x=w358, y=100.0) -> (x/y=w357:dbl)
              n182 = Multiply(x=w357, y="% Duty Cycle") -> (x*y=w356:dbl)
              n183 = Less?(x=w356, y=10000) -> (x < y?=w362:bool)
              n184 = case shown="True" w362 {
                tunnel: [w364 w370] -> w361
                tunnel: w356 -> [w365 w367]
                frame False {
                  n185 = Number To Decimal String(number=w365, width (-)=5) -> (decimal integer string=w364:string)
                }
                frame True {
                  n186 = Less?(x=w367, y=1000) -> (x < y?=w368:bool)
                  n187 = case shown="True" w368 {
                    tunnel: [w371 w377] -> w370
                    tunnel: w367 -> [w373 w376]
                    frame False {
                      # "greater then 1000"
                      n188 = Number To Decimal String(number=w373, width (-)=4) -> (decimal integer string=w374:string)
                      n189 = Concatenate Strings("0", w374) -> (w371:string)
                    }
                    frame True {
                      # "999"
                      n190 = Less?(x=w376, y=100) -> (x < y?=w379:bool)
                      n191 = case shown="True" w379 {
                        tunnel: [w380 w385] -> w377
                        tunnel: w376 -> [w383 w386]
                        frame False {
                          w381 = "0"
                          # "100 - 999"
                          # ">=100 <1000"
                          n192 = Number To Decimal String(number=w383, width (-)=3) -> (decimal integer string=w382:string)
                          n193 = Concatenate Strings(w381, w381, w382) -> (w380:string)
                        }
                        frame True {
                          n194 = Less?(x=w386, y=10) -> (x < y?=w388:bool)
                          n195 = case shown="True" w388 {
                            tunnel: w386 -> [w391 w395]
                            tunnel: [w389 w396] -> w385
                            frame False {
                              w390 = "0"
                              # "10 - 99"
                              # ">=10 but <100"
                              # "<100"
                              n196 = Number To Decimal String(number=w391, width (-)=2) -> (decimal integer string=w392:string)
                              n197 = Concatenate Strings(w390, w390, w390, w392) -> (w389:string)
                            }
                            frame True {
                              w394 = "0"
                              # "0-9"
                              # "<10"
                              n198 = Number To Decimal String(number=w395, width (-)=1) -> (decimal integer string=w397:string)
                              n199 = Concatenate Strings(w394, w394, w394, w394, w397) -> (w396:string)
                            }
                          }
                        }
                      }
                    }
                  }
                }
              }
              "Duty cycle" <- w361
              n200 = call "Simulate Signal"("Duty Cycle (%)"="% Duty Cycle", "Frequency"=w355, "Amplitude"=5.0) -> ("Square"=→"Waveform Graph":dynamicdata)  [unwired: 11 in, 1 out]
            }
            frame #6 {
              # "Period"
              # "Duty"
              n201 = local read "Select COM port"() -> (w399:refnum<visa-resource-name>)
              n202 = Concatenate Strings(w401, w400) -> (w402:string)
              n203 = VISA Write(VISA resource name=w399, write buffer=w402, error in (no error)=w404) -> (return count=→"T command Bytes sent":u32)  [unwired: 2 out]
            }
            frame #7 {
              n204 = Wait (ms)(milliseconds to wait=100) -> ()  [unwired: 1 out]
            }
            frame #8 {
              n205 = case shown="True" "Stop Button" {
                frame False {
                }
                frame True {
                  n206 = stacked-sequence {
                    frame #0 {
                      n207 = call "g_send.vi"("Input buffer size"=16384) -> ()  [unwired: 10 in, 1 out]
                    }
                    frame #1 {
                      n208 = Wait (ms)(milliseconds to wait=5) -> ()  [unwired: 1 out]
                    }
                    frame #2 {
                      n209 = local read "Select COM port"() -> (w409:refnum<visa-resource-name>)
                      n210 = VISA Close(VISA resource name=w409) -> ()  [unwired: 1 in, 1 out]
                    }
                    frame #3 {
                      n211 = Stop(stop? (T)=TRUE ("Stop? (T)")) -> ()
                    }
                  }
                }
              }
            }
          }
        }
      }
    }
    frame "R,C graphs" {
      n212 = stacked-sequence {
        frame #0 {
          # "Initialize communication"
          n213 = stacked-sequence {
            seq-local: [w416 _ _ _ _ _] -> [_ _ _ w432 _ w449]
            seq-local: [w413 _ _ _ _ _] -> [_ _ _ w431 _ w444]
            seq-local: [_ w425 _ _ _ _] -> [_ _ w429 _ _ _]
            frame #0 {
              w423 = 0
              # "Clear Board ID icon"
              n214 = local read "Select COM port"() -> (w411:refnum<visa-resource-name>)
              n215 = local read "baud rate"() -> (w412:u32)
              n216 = call "VISA Configure Serial Port (Instr)mod.vi"("VISA resource name"=w411, "Enable Termination\nChar (T)"=FALSE, "baud rate (9600)"=w412, "data bits (8)"=8, "parity (0:none)"=w423, "flow control (0:none)"=w423) -> ("VISA resource name out"=w419:refnum<visa-resource-name>, "Name"=w415:string, "error out"=w420:errorcluster)  [unwired: 6 in, 1 out]
              n217 = VISA Open(error in (no error)=w420, VISA resource name=w419) -> (VISA resource name=w421:refnum<visa-resource-name>, error out=w422:errorcluster)  [unwired: 3 out]
              n218 = local write "Message"("") -> ()
              n219 = local write "Connected to:"(w415) -> ()
              n220 = VISA Flush I/O Buffer(VISA resource name=w421, mask (16)=u16 16 ("Maskieren (16)"), error in (no error)=w422) -> (VISA resource name out=w413:refnum<visa-resource-name>, error out=w416:errorcluster)
            }
            frame #1 {
              n221 = call "No_COM_port_found_EXIT.vi"("Message In"="No COM port found") -> ("STOP"=w425:bool, "Message Out"=w427:string, "COM PORTS"=w426:string[])  [unwired: 6 in, 2 out]
              n222 = local write "Message"(w427) -> ()
              n223 = local write "Available COM ports"(w426) -> ()
            }
            frame #2 {
              n224 = Stop(stop? (T)=w429) -> ()
            }
            frame #3 {
              w436 = u16 16  # I/O Receive Buffer mask
              # "Request board ID\nchar. sent \"i\""
              # "Request Board ID"
              # "Flushes and discards \ncontents of the \nreceive buffer"
              n225 = local read "Input buffer size"() -> (w430:u32)
              n226 = Concatenate Strings("i", "\r") -> (w434:string)
              n227 = VISA Set I/O Buffer Size(VISA resource name=w431, mask (16)=w436, size (4096)=w430, error in (no error)=w432) -> (VISA resource name out=w438:refnum<visa-resource-name>, error out=w437:errorcluster)
              n228 = VISA Flush I/O Buffer(VISA resource name=w438, mask (16)=w436, error in (no error)=w437) -> (VISA resource name out=w440:refnum<visa-resource-name>, error out=w439:errorcluster)
              n229 = VISA Write(VISA resource name=w440, write buffer=w434, error in (no error)=w439) -> ()  [unwired: 3 out]
            }
            frame #4 {
              n230 = Wait (ms)(milliseconds to wait=100) -> ()  [unwired: 1 out]
            }
            frame #5 {
              # "Will be true if there is no reply from\nthe unit"
              # "Unit replies with the board ID"
              n231 = property class="Instr"(reference=w444) -> (reference out=w445:refnum<visa-resource-name>, "Bytes at Port"=w447:u32)  [unwired: 1 in, 1 out]
              n232 = Less Or Equal?(x=w447, y=1) -> (x <= y?=w450:bool)
              n233 = case shown="False" w450 {
                tunnel: w449 -> [w452 w455]
                tunnel: [w452 w454] -> w448
                tunnel: w445 -> [_ w453]
                frame False {
                  # "RESET USB = GREEN"
                  n234 = local write "RESET USB"(FALSE) -> ()
                }
                frame True {
                  n235 = stacked-sequence {
                    tunnel: w455 -> [w458 _ _]
                    tunnel: [w457 _ _] -> w454
                    tunnel: w453 -> [w456 _ _]
                    frame #0 {
                      # "Close VISA"
                      n236 = VISA Close(VISA resource name=w456, error in (no error)=w458) -> (error out=w457:errorcluster)
                    }
                    frame #1 {
                      # "REST USB = RED"
                      n237 = local write "RESET USB"(TRUE) -> ()
                    }
                    frame #2 {
                      n238 = Stop(stop? (T)=TRUE ("Stop? (T)")) -> ()
                    }
                  }
                }
              }
              n239 = VISA Read(VISA resource name=w445, byte count=w447, error in (no error)=w448) -> (read buffer=w443:string, return count=w442:u32)  [unwired: 2 out]
              n240 = local write "Actual bytes read"(w442) -> ()
              n241 = local write "Message"(w443) -> ()
            }
          }
        }
        frame #1 {
          n242 = while {
            stop <- w462 stop-if-true
            n243 = stacked-sequence {
              seq-local: [w464 _ _ _ _ _ _ _ _ _ _ _] -> [_ _ w472 _ _ _ _ _ _ _ _ _]
              seq-local: [_ _ _ _ w482 _ _ _ _ _ _ _] -> [_ _ _ _ _ _ _ w502 w505 _ _ _]
              seq-local: [_ _ w471 _ _ _ _ _ _ _ _ _] -> [_ _ _ _ w480 _ _ _ _ _ _ _]
              seq-local: [_ _ _ _ w479 _ _ _ _ _ _ _] -> [_ _ _ _ _ _ w494 _ _ _ _ _]
              seq-local: [_ _ _ _ _ _ w493 _ _ _ _ _] -> [_ _ _ _ _ _ _ _ _ _ _ _]
              frame #0 {
                # "Get into case 18 in the \"Communication protocol.\" Both capacitance and resistance measurements started by the same case 18."
                n244 = local read "Select COM port"() -> (w465:refnum<visa-resource-name>)
                n245 = Concatenate Strings("C", "\r") -> (w466:string)
                n246 = VISA Write(VISA resource name=w465, write buffer=w466) -> (error out=w464:errorcluster)  [unwired: 1 in, 2 out]
              }
              frame #1 {
                n247 = Wait (ms)(milliseconds to wait=50) -> ()  [unwired: 1 out]
              }
              frame #2 {
                # "Reply from CNK : \"Capacitance and resistance test, waiting for your input.\""
                n248 = local read "Select COM port"() -> (w470:refnum<visa-resource-name>)
                n249 = property class="Instr"(reference=w470, error in=w472) -> (reference out=w475:refnum<visa-resource-name>, error out=w471:errorcluster, "Bytes at Port"=w474:u32)
                n250 = local write "Bytes at Port"(w474) -> ()
                n251 = VISA Read(VISA resource name=w475, byte count=w474) -> (read buffer=w473:string)  [unwired: 1 in, 3 out]
                n252 = local write "Message"(w473) -> ()
              }
              frame #3 {
                n253 = while {
                  stop <- "Apply current setting" stop-if-true
                }
              }
              frame #4 {
                w477 = ""
                # "Ring selector:\n0 - Select graph\n1 - Select numeric capacitance"
                n254 = case shown="7" "Ring" {
                  tunnel: ["5" "3" "6" "a" "b" "c" "d" "e"] -> w482
                  frame 0, Default {
                    # "C Graph"
                  }
                  frame 1 {
                    # "C numeric"
                  }
                  frame 2 {
                    # "flags = 6"
                    # "Call resistance test"
                  }
                  frame 3 {
                  }
                  frame 4 {
                  }
                  frame 5 {
                  }
                  frame 6 {
                  }
                  frame 7 {
                  }
                }
                n255 = local read "Select COM port"() -> (w478:refnum<visa-resource-name>)
                n256 = VISA Write(VISA resource name=w478, write buffer=w482, error in (no error)=w480) -> (error out=w479:errorcluster)  [unwired: 2 out]
                n257 = local write "Message"(w477) -> ()
                n258 = local write "Units"(w477) -> ()
              }
              frame #5 {
                n259 = Wait (ms)(milliseconds to wait=50) -> ()  [unwired: 1 out]
              }
              frame #6 {
                # "Read text message sent from CNK\nThis message is sent from communication protocol"
                n260 = case shown="True" TRUE {
                  tunnel: w494 -> [w495 w498]
                  tunnel: [w495 w497] -> w493
                  frame False {
                  }
                  frame True {
                    n261 = local read "Select COM port"() -> (w496:refnum<visa-resource-name>)
                    n262 = property class="Instr"(reference=w496, error in=w498) -> (reference out=w501:refnum<visa-resource-name>, error out=w497:errorcluster, "Bytes at Port"=w500:u32)
                    n263 = local write "Bytes at Port"(w500) -> ()
                    n264 = VISA Read(VISA resource name=w501, byte count=w500) -> (read buffer=w499:string)  [unwired: 1 in, 3 out]
                    n265 = local write "Message"(w499) -> ()
                  }
                }
              }
              frame #7 {
                n266 = case shown="\"False\", Default" w502 {
                  frame "False", Default {
                    n267 = Wait (ms)(milliseconds to wait=20000) -> ()  [unwired: 1 out]
                  }
                  frame "a", "b", "c", "d", "e" {
                    n268 = Wait (ms)(milliseconds to wait=3000) -> ()  [unwired: 1 out]
                  }
                }
              }
              frame #8 {
                n269 = case shown="\"6\", \"a\", \"b\", \"c\", \"d\", \"e\"" w505 {
                  frame "3", Default {
                    n270 = local read "Select COM port"() -> (w510:refnum<visa-resource-name>)
                    n271 = property class="Instr"(reference=w510) -> (reference out=w508:refnum<visa-resource-name>, error out=w525:errorcluster, "Bytes at Port"=w509:u32)  [unwired: 1 in]
                    n272 = local write "Bytes at Port"(w509) -> ()
                    n273 = call "Exit_prog.vi"("EN/DIS"=TRUE, "error in (no error)"=w525, "USB Interface Name"=w510) -> ("error out"=w524:errorcluster)  [unwired: 6 in, 2 out]
                    n274 = VISA Read(VISA resource name=w508, byte count=w509, error in (no error)=w524) -> (read buffer=w523:string, return count=w512:u32)  [unwired: 2 out]
                    n275 = Divide(x=w512, y=6) -> (x/y=w521:dbl)
                    n276 = local write "Number of Samples"(w521) -> ()
                    n277 = local write "Actual bytes read"(w512) -> ()
                    n278 = String To Byte Array(string=w523) -> (unsigned byte array=w520:u8[])
                    n279 = Delete From Array(array=w520, length=32, index=0) -> (array with subset deleted=w519:u8[])  [unwired: 1 out]
                    n280 = call "U8_3_byte_Array_to_voltage_current_Rev03.vi"("Nmbr_of_datapoints"=w512, "Array In"=w519, "Div INPUT 2R"=1.0, "Div INPUT 1L"=1.0, "Shift INPUT 2R"=0.0, "Shift INPUT 1L"=0.0) -> ("INPUT 2R"=w507:dbl[])  [unwired: 6 in, 7 out]
                    n281 = call "Convert to Dynamic Data7"("Array"=w507) -> ("Dynamic Data Type"=w506:dynamicdata)  [unwired: 3 in]
                    n282 = local write "Resistance Test"(w506) -> ()
                  }
                  frame "5" {
                    (unwired) 0.0
                    # "Enable CH1"
                    # "Capacitance test is on CH1"
                    n283 = local read "Select COM port"() -> (w526:refnum<visa-resource-name>)
                    n284 = property class="Instr"(reference=w526) -> (reference out=w548:refnum<visa-resource-name>, error out=w547:errorcluster, "Bytes at Port"=w543:u32)  [unwired: 1 in]
                    n285 = local write "Bytes at Port"(w543) -> ()
                    n286 = call "Exit_prog.vi"("EN/DIS"=TRUE, "error in (no error)"=w547, "Bytes to read"=w543) -> ("error out"=w546:errorcluster, "RESET USB"=w544:bool)  [unwired: 6 in, 1 out]
                    n287 = VISA Read(VISA resource name=w548, byte count=w543, error in (no error)=w546) -> (read buffer=w545:string, return count=w542:u32)  [unwired: 2 out]
                    n288 = Divide(x=w542, y=6) -> (x/y=w540:dbl)
                    n289 = local write "Number of Samples"(w540) -> ()
                    n290 = local write "Actual bytes read"(w542) -> ()
                    n291 = local write "RESET USB"(w544) -> ()
                    n292 = String To Byte Array(string=w545) -> (unsigned byte array=w527:u8[])
                    n293 = call "U8_3_byte_Array_to_voltage_current_Rev03.vi"("Nmbr_of_datapoints"=w542, "Array In"=w527, "INPUT1 AC couple"=FALSE, "INPUT2 AC couple"=FALSE, "Div INPUT 2R"=1.0, "Div INPUT 1L"=1.0, "Shift INPUT 2R"=0.0, "AC/DC"=FALSE, "Shift INPUT 1L"=0.0) -> ("INPUT 1L"=w528:dbl[], "INPUT 2R"=w529:dbl[])  [unwired: 3 in, 6 out]
                    n294 = call "Input selector.vi"("Voltage INPUT2"=w529, "Voltage INPUT1"=w528, "Ring"=0) -> ("Sig Out"=→"VCH1":dynamicdata)  [unwired: 3 in, 5 out]
                  }
                  frame "6", "a", "b", "c", "d", "e" {
                    # "Resistance test"
                    n295 = local read "Select COM port"() -> (w562:refnum<visa-resource-name>)
                    n296 = property class="Instr"(reference=w562) -> (reference out=w575:refnum<visa-resource-name>, error out=w574:errorcluster, "Bytes at Port"=w570:u32)  [unwired: 1 in]
                    n297 = local write "Bytes at Port"(w570) -> ()
                    n298 = call "Exit_prog.vi"("EN/DIS"=TRUE, "error in (no error)"=w574, "Bytes to read"=w570, "USB Interface Name"=w562) -> ("error out"=w573:errorcluster, "RESET USB"=w571:bool)  [unwired: 5 in, 1 out]
                    n299 = VISA Read(VISA resource name=w575, byte count=w570, error in (no error)=w573) -> (read buffer=w572:string, return count=w556:u32)  [unwired: 2 out]
                    n300 = local write "RESET USB"(w571) -> ()
                    n301 = Divide(x=w556, y=6) -> (x/y=w568:dbl)
                    n302 = local write "Number of Samples"(w568) -> ()
                    n303 = String To Byte Array(string=w572) -> (unsigned byte array=w567:u8[])
                    n304 = local write "Actual bytes read"(w556) -> ()
                    n305 = Delete From Array(array=w567, length=32, index=0) -> (deleted portion=w561:u8[], array with subset deleted=w566:u8[])
                    n306 = Byte Array To String(unsigned byte array=w561) -> (string=w563:string)
                    n307 = local write "Message"(w563) -> ()
                    n308 = call "U8_3_byte_Array_to_voltage_current_Rev03.vi"("Nmbr_of_datapoints"=w556, "Array In"=w566, "Div INPUT 2R"=1.0, "Div INPUT 1L"=1.0, "Shift INPUT 2R"=0.0, "Shift INPUT 1L"=0.0) -> ("INPUT2 Vave"=→"CH1 Vave":dbl, "INPUT 1L"=w553:dbl[], "INPUT 2R"=w551:dbl[])  [unwired: 6 in, 5 out]
                    n309 = call "Convert to Dynamic Data6"("Array"=w551) -> ("Dynamic Data Type"=w550:dynamicdata)  [unwired: 3 in]
                    n310 = call "Convert to Dynamic Data5"("Array"=w553) -> ("Dynamic Data Type"=w552:dynamicdata)  [unwired: 3 in]
                    n311 = Merge Signals(w552, w550) -> (→"Resistance Test":dynamicdata)
                  }
                }
              }
              frame #9 {
                n312 = Wait (ms)(milliseconds to wait=300) -> ()  [unwired: 1 out]
              }
              frame #10 {
                n313 = local read "Message"() -> (w577:string)
                n314 = case shown="\"Resistance Range is 17 to 170   \"" w577 {
                  frame "Resistance Range is 170k to 1.7M", Default {
                    # "kOhm"
                    n315 = local read "CH1 Vave"() -> (w580:dbl)
                    n316 = formula code="RUT = (4400000 - current_val*10**6) * 27 / (current_val*10**6);"("current_val"=w580) -> ("RUT"=w579:dbl)
                    n317 = local write "Units"("kOhm") -> ()
                    n318 = local write "Resistance"(w579) -> ()
                  }
                  frame "Resistance Range is 1.7k to 17k " {
                    # "Ohm"
                    n319 = local read "CH1 Vave"() -> (w583:dbl)
                    n320 = formula code="RUT = (4400000 - current_val*10**6) * 270 / (current_val*10**6);"("current_val"=w583) -> ("RUT"=w582:dbl)
                    n321 = local write "Resistance"(w582) -> ()
                    "Units" <- "Ohm"
                  }
                  frame "Resistance Range is 17 to 170   " {
                    # "Ohm"
                    # "current_val = ((4400000 - current_val) * 27 / (current_val/100);"
                    n322 = local read "CH1 Vave"() -> (w586:dbl)
                    n323 = formula code="RUT = (4400000 - current_val*10**6) * 27 / (current_val*10**6/100);"("current_val"=w586) -> ("RUT"=→"Resistance":dbl)
                    n324 = local write "Units"("Ohm") -> ()
                  }
                  frame "Resistance Range is 17k to 170k" {
                    # "Ohm"
                    n325 = local read "CH1 Vave"() -> (w589:dbl)
                    n326 = formula code="RUT = ((4400000 - current_val*10**6) * 2700)/ (current_val*10**6);"("current_val"=w589) -> ("RUT"=w588:dbl)
                    n327 = local write "Units"("Ohm") -> ()
                    n328 = local write "Resistance"(w588) -> ()
                  }
                  frame "Resistance Range is 1.7M to 17M" {
                    n329 = local read "CH1 Vave"() -> (w591:dbl)
                    n330 = formula code="RUT = ((4400000 - current_val*10**6) * 2700)/ (current_val*10**6);"("current_val"=w591) -> ("RUT"=w590:dbl)
                    n331 = local write "Units"("Ohm") -> ()
                    n332 = local write "Resistance"(w590) -> ()
                  }
                }
              }
              frame #11 {
                n333 = local read "Select COM port"() -> (w594:refnum<visa-resource-name>)
                n334 = call "STOP.vi"("stop"=TRUE, "Select COM port"=w594) -> ()  [unwired: 9 in, 1 out]
              }
            }
            n335 = local read "Select COM port"() -> (w461:refnum<visa-resource-name>)
            n336 = call "STOP.vi"("stop"="Exit", "Select COM port"=w461) -> ("False"=w462:bool)  [unwired: 9 in]
          }
        }
      }
    }
    frame "Datalogger" {
      # "How to determine if read can be done based on the number of bytes at the port"
      n337 = stacked-sequence {
        frame #0 {
          # "Initialize communication"
          n338 = stacked-sequence {
            seq-local: [_ _ w606 _ _ _] -> [_ _ _ w623 _ w640]
            seq-local: [_ _ _ w621 _ _] -> [_ _ _ _ _ _]
            seq-local: [w595 _ _ _ _ _] -> [_ w599 _ _ _ _]
            frame #0 {
              n339 = call "No_COM_port_found_EXIT.vi"("Message In"="No COM port found") -> ("STOP"=w595:bool, "Message Out"=w596:string, "COM PORTS"=w597:string[])  [unwired: 6 in, 2 out]
              n340 = local write "Message"(w596) -> ()
              n341 = local write "Available COM ports"(w597) -> ()
            }
            frame #1 {
              n342 = Stop(stop? (T)=w599) -> ()
            }
            frame #2 {
              w615 = 0
              # "Clear Board ID icon"
              n343 = local read "Select COM port"() -> (w600:refnum<visa-resource-name>)
              n344 = String To Byte Array(string=w600) -> (unsigned byte array=w609:u8[])
              n345 = Index Array(array=w609, index=0) -> ()  [unwired: 1 out]
              n346 = local read "baud rate"() -> (w605:u32)
              n347 = case shown="False" FALSE {
                tunnel: ["" "Select another COM"] -> w603
                frame False {
                }
                frame True {
                }
              }
              n348 = call "VISA Configure Serial Port (Instr)mod.vi"("VISA resource name"=w600, "Enable Termination\nChar (T)"=FALSE, "baud rate (9600)"=w605, "data bits (8)"=8, "parity (0:none)"=w615, "flow control (0:none)"=w615) -> ("VISA resource name out"=w611:refnum<visa-resource-name>, "Name"=w604:string, "error out"=w612:errorcluster)  [unwired: 6 in, 1 out]
              n349 = VISA Open(error in (no error)=w612, VISA resource name=w611) -> (VISA resource name=w613:refnum<visa-resource-name>, error out=w614:errorcluster)  [unwired: 3 out]
              n350 = local write "Connected to:"(w604) -> ()
              n351 = VISA Flush I/O Buffer(VISA resource name=w613, mask (16)=u16 16 ("Maskieren (16)"), error in (no error)=w614) -> (error out=w606:errorcluster)  [unwired: 1 out]
              n352 = local write "Message"(w603) -> ()
              n353 = local write "Message"("") -> ()
            }
            frame #3 {
              w626 = u16 16  # I/O Receive Buffer mask
              # "Sets buffer size"
              # "16384 bytes long"
              # "Request board ID\nchar. sent \"i\""
              # "Request Board ID"
              # "Flushes and discards \ncontents of the \nreceive buffer"
              n354 = local read "Select COM port"() -> (w620:refnum<visa-resource-name>)
              n355 = local read "Input buffer size"() -> (w622:u32)
              n356 = Concatenate Strings("i", "\r") -> (w625:string)
              n357 = VISA Set I/O Buffer Size(VISA resource name=w620, mask (16)=w626, size (4096)=w622, error in (no error)=w623) -> (VISA resource name out=w628:refnum<visa-resource-name>, error out=w627:errorcluster)
              n358 = VISA Flush I/O Buffer(VISA resource name=w628, mask (16)=w626, error in (no error)=w627) -> (VISA resource name out=w630:refnum<visa-resource-name>, error out=w629:errorcluster)
              n359 = VISA Write(VISA resource name=w630, write buffer=w625, error in (no error)=w629) -> (error out=w621:errorcluster)  [unwired: 2 out]
            }
            frame #4 {
              n360 = Wait (ms)(milliseconds to wait=100) -> ()  [unwired: 1 out]
            }
            frame #5 {
              # "Will be true if there is no reply from\nthe unit"
              # "Unit replies with the board ID"
              n361 = local read "Select COM port"() -> (w632:refnum<visa-resource-name>)
              n362 = property class="Instr"(reference=w632) -> (reference out=w636:refnum<visa-resource-name>, "Bytes at Port"=w638:u32)  [unwired: 1 in, 1 out]
              n363 = Less Or Equal?(x=w638, y=1) -> (x <= y?=w641:bool)
              n364 = case shown="False" w641 {
                tunnel: w640 -> [w643 w646]
                tunnel: [w643 w645] -> w639
                tunnel: w636 -> [_ w644]
                frame False {
                  # "RESET USB = GREEN"
                  n365 = local write "RESET USB"(FALSE) -> ()
                }
                frame True {
                  n366 = stacked-sequence {
                    tunnel: w646 -> [w649 _ _]
                    tunnel: [w648 _ _] -> w645
                    tunnel: w644 -> [w647 _ _]
                    frame #0 {
                      # "Close VISA"
                      n367 = VISA Close(VISA resource name=w647, error in (no error)=w649) -> (error out=w648:errorcluster)
                    }
                    frame #1 {
                      # "REST USB = RED"
                      n368 = local write "RESET USB"(TRUE) -> ()
                    }
                    frame #2 {
                      n369 = Stop(stop? (T)=TRUE ("Stop? (T)")) -> ()
                    }
                  }
                }
              }
              n370 = VISA Read(VISA resource name=w636, byte count=w638, error in (no error)=w639) -> (read buffer=w635:string, return count=w634:u32)  [unwired: 2 out]
              n371 = local write "Message"(w635) -> ()
              n372 = local write "Actual bytes read"(w634) -> ()
              n373 = Get Date/Time In Seconds() -> (seconds since 1Jan1904=→"Current time":timestamp)
            }
          }
        }
        frame #1 {
          n374 = while {
            stop <- w655 stop-if-true
            w655 = FALSE
            # "to the next frame"
            n375 = stacked-sequence {
              seq-local: [w656 _ _ _ _ _] -> [_ w678 _ w682 w720 w738]
              seq-local: [_ w677 _ _ _ _] -> [_ _ _ w683 w719 _]
              seq-local: [_ _ _ _ _ w761] -> [_ _ _ _ _ _]
              seq-local: [_ _ _ _ w722 _] -> [_ _ _ _ _ w760]
              seq-local: [_ _ _ _ w721 _] -> [_ _ _ _ _ w759]
              tunnel: [_ _ _ _ w718 _] -> w652
              frame #0 {
                n376 = while {
                  tunnel: [w661] -> w656
                  stop <- w657 stop-if-true
                  n377 = case shown="4" "Function Select" {
                    tunnel: ["a" "d" "z" "U" "c" "V"] -> w661
                    frame 0, Default {
                      # "Upload data"
                    }
                    frame 1 {
                      # "Erase data all sectors"
                    }
                    frame 2 {
                      # "'z'"
                      # "Write datalogger configuration"
                      # "Write datalogger config\nWhen z is sent MCU will wait for 4 characters. The first and second characters will be decoded into dividor values.\nByte 0 : Divider CH0\nByte 1 : Divider CH1\nByte 2 : Timer value character\nByte 3 : 'a' of 'b' - if 'a' Erase all data check mark is ON"
                    }
                    frame 3 {
                      # "Read memory address"
                    }
                    frame 4 {
                      # "Record data wth datalogger"
                    }
                    frame 5 {
                      # "When 'V' is sent to the instrument, CNK will write data into the volage and current buffers, send this data back to PC"
                      # "Write fake data"
                    }
                  }
                  n378 = case shown="True" "STOP" {
                    frame False {
                    }
                    frame True {
                      n379 = stacked-sequence {
                        frame #0 {
                          n380 = local read "Select COM port"() -> (w663:refnum<visa-resource-name>)
                          n381 = call "g_send.vi"("Input buffer size"=16384, "USB Interface Name"=w663) -> ()  [unwired: 9 in, 1 out]
                        }
                        frame #1 {
                          n382 = Wait (ms)(milliseconds to wait=5) -> ()  [unwired: 1 out]
                        }
                        frame #2 {
                          n383 = local read "Select COM port"() -> (w666:refnum<visa-resource-name>)
                          n384 = VISA Close(VISA resource name=w666) -> ()  [unwired: 1 in, 1 out]
                        }
                        frame #3 {
                          n385 = Stop(stop? (T)=TRUE ("Stop? (T)")) -> ()
                        }
                      }
                    }
                  }
                  n386 = And(x="Send Configuration", y="Apply") -> (x .and. y?=w657:bool)
                }
              }
              frame #1 {
                w674 = 0
                w676 = ""
                # "Clear windows"
                # "Menu selection"
                # "Send previously selected character to the MCU"
                n387 = local write "Data Read from memory HEX"(w676) -> ()
                n388 = local write "Bytes at Port"(w674) -> ()
                n389 = local write "Actual bytes read"(w674) -> ()
                n390 = local write "Memory Responce"(w676) -> ()
                n391 = local read "Select COM port"() -> (w675:refnum<visa-resource-name>)
                n392 = Concatenate Strings(w678, "\r") -> (w679:string)
                n393 = VISA Write(VISA resource name=w675, write buffer=w679) -> (error out=w677:errorcluster)  [unwired: 1 in, 2 out]
              }
              frame #2 {
                n394 = Wait (ms)(milliseconds to wait=100) -> ()  [unwired: 1 out]
              }
              frame #3 {
                # "Menu selection"
                n395 = case shown="\"z\"" w682 {
                  tunnel: w683 -> [_ w684 _ w690 _ _]
                  frame "a", Default {
                    # "Get recorded data"
                  }
                  frame "U" {
                    n396 = flat-sequence {
                      tunnel: w684 -> [w686]
                      frame #0 {
                        n397 = local read "Select COM port"() -> (w685:refnum<visa-resource-name>)
                        n398 = VISA Write(VISA resource name=w685, write buffer="Enter mem address in 5 decimal values. Example: 06142", error in (no error)=w686) -> ()  [unwired: 3 out]
                      }
                      frame #1 {
                        n399 = Wait (ms)(milliseconds to wait=10) -> ()  [unwired: 1 out]
                      }
                    }
                  }
                  frame "V" {
                    # "When 'V' is sent to the instrument, CNK will write data into the volage and current buffers, send this data back to PC"
                    n400 = Wait (ms)(milliseconds to wait=2000) -> ()  [unwired: 1 out]
                  }
                  frame "z" {
                    # "Write datalogger configuration"
                    n401 = stacked-sequence {
                      seq-local: [w691 _ _ _] -> [_ _ w708 _]
                      tunnel: w690 -> [w693 _ _ _]
                      frame #0 {
                        # "Send 2 bytes"
                        # "dividorCH1 = buff[1];"
                        # "dividorCH0 = buff[0];"
                        # "Character 'z' will set MCU to wait for configuration data. Currently a maximum of 2 characters can be sent."
                        n402 = case shown="1" "Voltage Range CH1" {
                          tunnel: ["1" "2" "3" "4"] -> w697
                          frame 0, Default {
                            # "MCU will set dividor to 1"
                          }
                          frame 1 {
                            # "MCU will set dividor to51"
                          }
                          frame 2 {
                            # "MCU will set dividor to 80"
                          }
                          frame 3 {
                            # "MCU will set dividor to10"
                          }
                        }
                        n403 = case shown="0, Default" "Voltage Range CH0" {
                          tunnel: ["1" "2" "3" "4"] -> w698
                          frame 0, Default {
                            # "MCU will set dividor to 1"
                          }
                          frame 1 {
                            # "51"
                          }
                          frame 2 {
                            # "80"
                          }
                          frame 3 {
                            # "10"
                          }
                        }
                        n404 = local read "Select COM port"() -> (w692:refnum<visa-resource-name>)
                        n405 = Concatenate Strings(w698, w697) -> (w694:string)
                        n406 = VISA Write(VISA resource name=w692, write buffer=w694, error in (no error)=w693) -> (error out=w691:errorcluster)  [unwired: 2 out]
                      }
                      frame #1 {
                        n407 = Wait (ms)(milliseconds to wait=100) -> ()  [unwired: 1 out]
                      }
                      frame #2 {
                        n408 = local read "Select COM port"() -> (w713:refnum<visa-resource-name>)
                        n409 = case shown="True" "Erase All Data?" {
                          tunnel: ["b" "a"] -> w710
                          frame False {
                          }
                          frame True {
                          }
                        }
                        n410 = Concatenate Strings("Time Interval 0-9 sec", w710) -> (w712:string)
                        n411 = VISA Write(VISA resource name=w713, write buffer=w712, error in (no error)=w708) -> ()  [unwired: 3 out]
                      }
                      frame #3 {
                        n412 = Wait (ms)(milliseconds to wait=10000) -> ()  [unwired: 1 out]
                      }
                    }
                  }
                  frame "d " {
                    # "Memory sector eraze"
                  }
                  frame "c" {
                    n413 = Wait (ms)(milliseconds to wait=10) -> ()  [unwired: 1 out]
                  }
                }
              }
              frame #4 {
                # "Waiting for CNK responce"
                n414 = while {
                  tunnel: w719 -> [w726]
                  tunnel: [w729] -> w722
                  tunnel: [w727] -> w721
                  tunnel: w720 -> [w728]
                  tunnel: [w723] -> w718
                  stop <- w724 stop-if-true
                  # "If config is downloaded exit from"
                  n415 = local read "Select COM port"() -> (w725:refnum<visa-resource-name>)
                  n416 = property class="Instr"(reference=w725, error in=w726) -> (error out=w729:errorcluster, "Bytes at Port"=w727:u32)  [unwired: 1 out]
                  n417 = local write "Bytes at Port"(w727) -> ()
                  n418 = case shown="\"c\"" w728 {
                    tunnel: [12 0 10 25 20 4] -> w723
                    frame "d" {
                    }
                    frame "a", Default {
                    }
                    frame "V" {
                    }
                    frame "z" {
                      # "Reply with \"Configuration is downloaded\""
                      # "Config send"
                    }
                    frame "c" {
                    }
                    frame "U" {
                    }
                  }
                  n419 = Greater?(x=w727, y=w723) -> (0:w724:bool)
                }
              }
              frame #5 {
                w768 = 0.0
                # "The second byte sent back is div CH1"
                # "The first byte sent back is div CH0"
                # "Each sample is 3 bytes long"
                # "This is the responce to \"Download Configuration\" command. \nThe first 26 bytes is text \"Configuration is downloaded\". This data stream has any sence only when a new configuration is downloaded."
                # "0xFFFFFF is converter to  -93nV. 0xFFFFFF is one step on A/D converter"
                n420 = Equal?(x=w738, y="V") -> (x = y?=w747:bool)
                n421 = Equal?(x=w738, y="z") -> (x = y?=w748:bool)
                n422 = Equal?(x=w738, y="c") -> (x = y?=w736:bool)
                n423 = Or(x=w747, y=w748) -> (x .or. y?=w739:bool)
                n424 = Or(x=w739, y=w736) -> (x .or. y?=w740:bool)
                n425 = local read "Select COM port"() -> (w746:refnum<visa-resource-name>)
                n426 = VISA Read(VISA resource name=w746, byte count=w759, error in (no error)=w760) -> (read buffer=w751:string, return count=w757:u32, error out=w761:errorcluster)  [unwired: 1 out]
                "Data Read from memory HEX" <- w751
                n427 = case shown="True" w740 {
                  tunnel: ["" w788] -> w745
                  tunnel: [w774 w787] -> w744
                  tunnel: [w773 w786] -> w743
                  tunnel: w751 -> [w775 w783]
                  tunnel: [w772 w779] -> w750
                  frame False {
                    w776 = 1
                    n428 = String Subset(string=w775, offset (0)=1, length (rest)=w776) -> (substring=w773:string)
                    n429 = String To Byte Array(string=w775) -> (unsigned byte array=w772:u8[])
                    n430 = String Subset(string=w775, offset (0)=0, length (rest)=w776) -> (substring=w774:string)
                  }
                  frame True {
                    w777 = 1
                    w778 = 0
                    n431 = Add(x=w778, y=w777) -> (x+y=w784:i32)
                    n432 = String To Byte Array(string=w783) -> (unsigned byte array=w782:u8[])
                    n433 = String Subset(string=w783, offset (0)=w784, length (rest)=w777) -> (substring=w786:string)
                    n434 = String Subset(string=w783, offset (0)=w778, length (rest)=w777) -> (substring=w787:string)
                    n435 = String Subset(string=w783, offset (0)=2, length (rest)=32) -> (substring=w788:string)
                    n436 = Delete From Array(array=w782, index=0) -> (array with subset deleted=w779:u8[])  [unwired: 1 in, 1 out]
                  }
                }
                "Memory Responce" <- w745
                "Divider CH0 Replied back" <- w744
                "Divider CH1 Replied back" <- w743
                n437 = Subtract(x=w757, y=2) -> (x-y=w755:u32)
                n438 = Divide(x=w755, y=3) -> (x/y=w754:dbl)
                n439 = local write "Actual bytes read"(w757) -> ()
                n440 = local write "Number of Samples"(w754) -> ()
                n441 = call "Datalogger_U8_3_byte_Array_to_voltage_current_Rev03.vi"("Nmbr_of_datapoints"=w754, "Array In"=w750, "CH1 Shift V"=w768, "AC/DC"=FALSE, "CH0 Shift V"=w768) -> ("CH0 multipler"=→"CH0 multiplier":dbl, "CH1 multipler"=→"CH1 multiplier":dbl, "Voltage"=w764:dbl[], "Current"=w765:dbl[])  [unwired: 10 in, 9 out]
                n442 = call "Convert to Dynamic Data2"("Array"=w764) -> ("Dynamic Data Type"=w763:dynamicdata)  [unwired: 3 in]
                n443 = call "Convert to Dynamic Data"("Array"=w765) -> ("Dynamic Data Type"=w762:dynamicdata)  [unwired: 3 in]
                n444 = property on="V data logger" class="WFGraph (strict)"("XScale.Maximum"="X-max 2", "XScale.Minimum"=w768) -> ()  [unwired: 2 in, 2 out]
                n445 = Merge Signals(w763, w762) -> (→"V data logger":dynamicdata)
              }
            }
            n446 = Equal?(x=w652, y=29) -> (x = y?=w654:bool)
            n447 = Or(x=w654, y=w655) -> ()  [unwired: 1 out]
          }
        }
      }
    }
    frame "Sensor" {
      # "How to determine if read can be done based on the number of bytes at the port"
      n448 = stacked-sequence {
        frame #0 {
          # "Initialize communication"
          n449 = stacked-sequence {
            seq-local: [w796 _ _ _] -> [_ w811 _ w827]
            seq-local: [w791 _ _ _] -> [_ w810 _ _]
            seq-local: [_ w808 _ _] -> [_ _ _ _]
            frame #0 {
              w804 = 0
              # "Clear Board ID icon"
              n450 = local read "Select COM port"() -> (w789:refnum<visa-resource-name>)
              n451 = Equal?(x=w789, y="COM3") -> (x = y?=w794:bool)
              n452 = local read "baud rate"() -> (w790:u32)
              n453 = Stop(stop? (T)=w794) -> ()
              n454 = case shown="True" w794 {
                tunnel: ["" "Select another COM"] -> w793
                frame False {
                }
                frame True {
                }
              }
              n455 = call "VISA Configure Serial Port (Instr)mod.vi"("VISA resource name"=w789, "Enable Termination\nChar (T)"=FALSE, "baud rate (9600)"=w790, "data bits (8)"=8, "parity (0:none)"=w804, "flow control (0:none)"=w804) -> ("VISA resource name out"=w800:refnum<visa-resource-name>, "Name"=w795:string, "error out"=w801:errorcluster)  [unwired: 6 in, 1 out]
              n456 = VISA Open(error in (no error)=w801, VISA resource name=w800) -> (VISA resource name=w802:refnum<visa-resource-name>, error out=w803:errorcluster)  [unwired: 3 out]
              n457 = local write "Connected to:"(w795) -> ()
              n458 = VISA Flush I/O Buffer(VISA resource name=w802, mask (16)=u16 16 ("Maskieren (16)"), error in (no error)=w803) -> (VISA resource name out=w791:refnum<visa-resource-name>, error out=w796:errorcluster)
              n459 = local write "Message"(w793) -> ()
              n460 = local write "Message"("") -> ()
            }
            frame #1 {
              w815 = u16 16  # I/O Receive Buffer mask
              # "Sets buffer size"
              # "16384 bytes long"
              # "Request board ID\nchar. sent \"i\""
              # "Request Board ID"
              # "Flushes and discards \ncontents of the \nreceive buffer"
              n461 = local read "Input buffer size"() -> (w809:u32)
              n462 = Concatenate Strings("i", "\r") -> (w813:string)
              n463 = VISA Set I/O Buffer Size(VISA resource name=w810, mask (16)=w815, size (4096)=w809, error in (no error)=w811) -> (VISA resource name out=w817:refnum<visa-resource-name>, error out=w816:errorcluster)
              n464 = VISA Flush I/O Buffer(VISA resource name=w817, mask (16)=w815, error in (no error)=w816) -> (VISA resource name out=w818:refnum<visa-resource-name>, error out=w808:errorcluster)
              n465 = VISA Write(VISA resource name=w818, write buffer=w813, error in (no error)=w808) -> ()  [unwired: 3 out]
            }
            frame #2 {
              n466 = Wait (ms)(milliseconds to wait=100) -> ()  [unwired: 1 out]
            }
            frame #3 {
              # "Will be true if there is no reply from\nthe unit"
              # "Unit replies with the board ID"
              n467 = local read "Select COM port"() -> (w820:refnum<visa-resource-name>)
              n468 = property class="Instr"(reference=w820) -> (reference out=w823:refnum<visa-resource-name>, "Bytes at Port"=w825:u32)  [unwired: 1 in, 1 out]
              n469 = Less Or Equal?(x=w825, y=1) -> (x <= y?=w828:bool)
              n470 = case shown="True" w828 {
                tunnel: w827 -> [w830 w833]
                tunnel: [w830 w832] -> w826
                tunnel: w823 -> [_ w831]
                frame False {
                  # "RESET USB = GREEN"
                  n471 = local write "RESET USB"(FALSE) -> ()
                }
                frame True {
                  n472 = stacked-sequence {
                    tunnel: w833 -> [w836 _ _]
                    tunnel: [w835 _ _] -> w832
                    tunnel: w831 -> [w834 _ _]
                    frame #0 {
                      # "Close VISA"
                      n473 = VISA Close(VISA resource name=w834, error in (no error)=w836) -> (error out=w835:errorcluster)
                    }
                    frame #1 {
                      # "REST USB = RED"
                      n474 = local write "RESET USB"(TRUE) -> ()
                    }
                    frame #2 {
                      n475 = Stop(stop? (T)=TRUE ("Stop? (T)")) -> ()
                    }
                  }
                }
              }
              n476 = VISA Read(VISA resource name=w823, byte count=w825, error in (no error)=w826) -> (read buffer=w822:string)  [unwired: 3 out]
              n477 = local write "Message"(w822) -> ()
              n478 = Get Date/Time In Seconds() -> (seconds since 1Jan1904=→"Current time 2":timestamp)
            }
          }
        }
        frame #1 {
          n479 = stacked-sequence {
            frame #0 {
              w841 = TRUE
              n480 = local read "Select COM port"() -> (w840:refnum<visa-resource-name>)
              n481 = call "CH0_Manual_range_select.vi"("Select COM port"=w840, "EN"=w841, "IN1 L"="Range select INPUT1 2") -> ()  [unwired: 8 in, 1 out]
              n482 = call "CH1_Manual_range_select.vi"("CH1"="Range select INPUT2 2", "EN"=w841, "Select COM port"=w840) -> ()  [unwired: 8 in, 1 out]
            }
            frame #1 {
              n483 = Stop(stop? (T)=TRUE) -> ()
            }
          }
        }
      }
    }
    frame "Cal" {
      n484 = stacked-sequence {
        frame #0 {
          n485 = stacked-sequence {
            seq-local: [w847 _ _ _ _ _ _] -> [_ _ w855 _ _ _ _]
            seq-local: [_ _ w854 _ _ _ _] -> [_ _ _ w867 _ _ _]
            seq-local: [_ _ _ w866 _ _ _] -> [_ _ _ _ _ w880 _]
            seq-local: [w845 _ _ _ _ _ _] -> [_ w849 _ _ _ _ _]
            frame #0 {
              # "Looking for available com ports"
              n486 = call "No_COM_port_found_EXIT.vi"("Message In"="No COM port found") -> ("STOP"=w845:bool, "Message Out"=w848:string, "COM PORTS"=w844:string[], "error out"=w847:errorcluster)  [unwired: 6 in, 1 out]
              n487 = local write "Message"(w848) -> ()
              n488 = local write "Available COM ports"(w844) -> ()
            }
            frame #1 {
              # "If no COM port is found exit the program"
              n489 = Stop(stop? (T)=w849) -> ()
            }
            frame #2 {
              w862 = 0
              n490 = local read "Select COM port"() -> (w853:refnum<visa-resource-name>)
              n491 = local read "baud rate"() -> (w850:u32)
              n492 = call "VISA Configure Serial Port (Instr)mod.vi"("VISA resource name"=w853, "Enable Termination\nChar (T)"=FALSE, "baud rate (9600)"=w850, "data bits (8)"=8, "parity (0:none)"=w862, "error in (no error)"=w855, "flow control (0:none)"=w862) -> ("VISA resource name out"=w858:refnum<visa-resource-name>, "Name"=w852:string, "Name 2"=w851:string, "error out"=w859:errorcluster)  [unwired: 5 in]
              n493 = local write "Connected to Name"(w851) -> ()
              n494 = VISA Open(error in (no error)=w859, VISA resource name=w858) -> (VISA resource name=w860:refnum<visa-resource-name>, error out=w861:errorcluster)  [unwired: 3 out]
              n495 = local write "Connected to:"(w852) -> ()
              n496 = VISA Flush I/O Buffer(VISA resource name=w860, mask (16)=u16 16 ("Maskieren (16)"), error in (no error)=w861) -> (error out=w854:errorcluster)  [unwired: 1 out]
            }
            frame #3 {
              w871 = u16 16  # I/O Receive Buffer mask
              # "Request board ID\nchar. sent \"i\""
              # "Send commend: Request Board ID. CNK will reply with a serial number"
              # "Flushes and discards \ncontents of the \nreceive buffer"
              n497 = local read "Input buffer size"() -> (w865:u32)
              n498 = local read "Select COM port"() -> (w864:refnum<visa-resource-name>)
              n499 = Concatenate Strings("i", "\r") -> (w869:string)
              n500 = VISA Set I/O Buffer Size(VISA resource name=w864, mask (16)=w871, size (4096)=w865, error in (no error)=w867) -> (VISA resource name out=w873:refnum<visa-resource-name>, error out=w872:errorcluster)
              n501 = VISA Flush I/O Buffer(VISA resource name=w873, mask (16)=w871, error in (no error)=w872) -> (VISA resource name out=w875:refnum<visa-resource-name>, error out=w874:errorcluster)
              n502 = VISA Write(VISA resource name=w875, write buffer=w869, error in (no error)=w874) -> (error out=w866:errorcluster)  [unwired: 2 out]
            }
            frame #4 {
              n503 = Wait (ms)(milliseconds to wait=400) -> ()  [unwired: 1 out]
            }
            frame #5 {
              # "If no responce exit application"
              n504 = local read "Select COM port"() -> (w878:refnum<visa-resource-name>)
              n505 = property class="Instr"(reference=w878, error in=w880) -> (reference out=w885:refnum<visa-resource-name>, error out=w879:errorcluster, "Bytes at Port"=w887:u32)
              n506 = Less Or Equal?(x=w887, y=1) -> (x <= y?=w888:bool)
              n507 = VISA Read(VISA resource name=w885, byte count=w887, error in (no error)=w879) -> (read buffer=w882:string, error out=w881:errorcluster)  [unwired: 2 out]
              n508 = case shown="True" w888 {
                tunnel: w885 -> [_ w893]
                tunnel: w881 -> [_ w892]
                frame False {
                  # "RESET USB = GREEN"
                  n509 = local write "RESET USB"(FALSE) -> ()
                }
                frame True {
                  n510 = stacked-sequence {
                    tunnel: w893 -> [w895 _ _]
                    tunnel: w892 -> [w894 _ _]
                    frame #0 {
                      # "Close VISA"
                      n511 = VISA Close(VISA resource name=w895, error in (no error)=w894) -> ()  [unwired: 1 out]
                    }
                    frame #1 {
                      # "REST USB = RED"
                      n512 = local write "RESET USB"(TRUE) -> ()
                    }
                    frame #2 {
                      n513 = Stop(stop? (T)=TRUE ("Stop? (T)")) -> ()
                    }
                  }
                }
              }
              n514 = Equal?(x=w882, y="") -> (x = y?=w883:bool)
              n515 = case shown="True" w883 {
                tunnel: [w889 "No Responce"] -> w877
                tunnel: w882 -> [w889 _]
                frame False {
                }
                frame True {
                }
              }
              n516 = local write "Message"(w877) -> ()
            }
            frame #6 {
              # "Once program responds with ID it returns to the main() to continue to collect data"
              n517 = Wait (ms)(milliseconds to wait=1000) -> ()  [unwired: 1 out]
            }
          }
        }
        frame #1 {
          n518 = stacked-sequence {
            seq-local: [w899 _ _ _ _ _] -> [_ w919 _ w928 _ _]
            seq-local: [_ w918 _ _ _ _] -> [_ _ _ _ _ _]
            frame #0 {
              n519 = while {
                tunnel: [w900] -> w899
                stop <- "Apply Memory Command" stop-if-true
                # "No data will be sent until Apply is pressed"
                n520 = case shown="12" "Memory Functions" {
                  tunnel: ["a" "d" "z" "U" "c" "2" "v" "D" "g" "A" "B" "E" "G"] -> w900
                  frame 0, Default {
                    # "Upload data"
                  }
                  frame 1 {
                    # "Erase data all sectors"
                  }
                  frame 2 {
                    # "'z'"
                    # "Write datalogger configuration"
                    # "When z is sent MCU will wait for 3 characters. The first and second characters will be decoded into dividor values."
                  }
                  frame 3 {
                    # "Read memory address"
                  }
                  frame 4 {
                    # "Record data wth datalogger"
                  }
                  frame 5 {
                    # "When 'V' is sent to the instrument, CNK will write data into the volage and current buffers, send this data back to PC"
                    # "Write fake data"
                  }
                  frame 6 {
                  }
                  frame 7 {
                  }
                  frame 8 {
                  }
                  frame 9 {
                    # "'A' Dial on PC for CH0 set to 1/1"
                  }
                  frame 10 {
                    # "'B' Dial on PC for CH0 set to 510k"
                  }
                  frame 11 {
                    # "'E' Dial on PC for CH0 set to 80.6k"
                  }
                  frame 12 {
                    # "'G' Dial on PC for CH0 set to 10k"
                  }
                }
              }
            }
            frame #1 {
              w920 = 0
              w922 = ""
              # "Clear windows"
              # "Menu selection"
              # "Send previously selected character to MCU"
              n521 = local read "Select COM port"() -> (w921:refnum<visa-resource-name>)
              n522 = Concatenate Strings(w919, "\r") -> (w923:string)
              n523 = local write "Data Read from memory HEX"(w922) -> ()
              n524 = local write "Memory Responce"(w922) -> ()
              n525 = VISA Write(VISA resource name=w921, write buffer=w923) -> (return count=w917:u32, error out=w918:errorcluster)  [unwired: 1 in, 1 out]
              n526 = local write "# of bytes written"(w917) -> ()
              n527 = local write "RESET USB"(FALSE) -> ()
              n528 = local write "Actual bytes read"(w920) -> ()
              n529 = local write "Bytes at Port"(w920) -> ()
            }
            frame #2 {
              n530 = Wait (ms)(milliseconds to wait=500) -> ()  [unwired: 1 out]
            }
            frame #3 {
              n531 = local read "Select COM port"() -> (w926:refnum<visa-resource-name>)
              n532 = property class="Instr"(reference=w926) -> (reference out=w931:refnum<visa-resource-name>, error out=w929:errorcluster, "Bytes at Port"=w930:u32)  [unwired: 1 in]
              n533 = VISA Read(VISA resource name=w931, byte count=w930, error in (no error)=w929) -> (read buffer=→"Reply":string)  [unwired: 3 out]
              n534 = case shown="\"D\"" w928 {
                selector: w928 -> [_ w938 _]
                tunnel: w926 -> [_ _ w939]
                frame "False", Default {
                }
                frame "D" {
                  n535 = call "divider_and_offset_Rev_03.vi"("Control Char"=w938) -> ("Div In1 Lft"=w937:dbl, "Div In2 Rgt"=w936:dbl, "INPUT2 shift sign"=w934:dbl, "INPUT1 shift sign"=w933:dbl, "Shift IN2 R ch1"=w932:dbl, "Shift IN1 L ch0"=w935:dbl)  [unwired: 6 in, 3 out]
                  n536 = local write "Divider INPUT2 R"(w937) -> ()
                  n537 = local write "Divider INPUT1 L"(w936) -> ()
                  n538 = local write "INPUT2 shift sign"(w934) -> ()
                  n539 = local write "Shift INPUT2 R"(w932) -> ()
                  n540 = local write "Shift INPUT1 L"(w935) -> ()
                  n541 = local write "INPU1 shift sign"(w933) -> ()
                }
                frame "A", "B", "E", "G" {
                  # "'A' Dial on PC for CH0 set to 1/1"
                  n542 = flat-sequence {
                    tunnel: w939 -> [_]
                    frame #0 {
                    }
                    frame #1 {
                      n543 = while {
                        stop <- "Stop Manual Range Select" stop-if-true
                        # "View Results on the LCD"
                      }
                    }
                  }
                }
              }
            }
            frame #4 {
              n544 = Wait (ms)(milliseconds to wait=1000) -> ()  [unwired: 1 out]
            }
            frame #5 {
              n545 = case shown="True" TRUE {
                frame False {
                }
                frame True {
                  n546 = stacked-sequence {
                    frame #0 {
                      n547 = local read "Select COM port"() -> (w943:refnum<visa-resource-name>)
                      n548 = call "g_send.vi"("Input buffer size"=16384, "USB Interface Name"=w943) -> ()  [unwired: 9 in, 1 out]
                    }
                    frame #1 {
                      n549 = Wait (ms)(milliseconds to wait=5) -> ()  [unwired: 1 out]
                    }
                    frame #2 {
                      n550 = local read "Select COM port"() -> (w946:refnum<visa-resource-name>)
                      n551 = VISA Close(VISA resource name=w946) -> ()  [unwired: 1 in, 1 out]
                    }
                    frame #3 {
                      n552 = Stop(stop? (T)=TRUE ("Stop? (T)")) -> ()
                    }
                  }
                }
              }
            }
          }
        }
      }
    }
    frame "Digital Sniffer" {
      n553 = stacked-sequence {
        frame #0 {
          n554 = stacked-sequence {
            seq-local: [w951 _ _ _ _ _ _] -> [_ _ w957 _ _ _ _]
            seq-local: [_ _ w956 _ _ _ _] -> [_ _ _ w967 _ _ _]
            seq-local: [_ _ _ w966 _ _ _] -> [_ _ _ _ _ w981 _]
            seq-local: [w949 _ _ _ _ _ _] -> [_ w953 _ _ _ _ _]
            frame #0 {
              # "Looking for available com ports"
              n555 = call "No_COM_port_found_EXIT.vi"("Message In"="No COM port found") -> ("STOP"=w949:bool, "Message Out"=w952:string, "COM PORTS"=w948:string[], "error out"=w951:errorcluster)  [unwired: 6 in, 1 out]
              n556 = local write "Message"(w952) -> ()
              n557 = local write "Available COM ports"(w948) -> ()
            }
            frame #1 {
              # "If no COM port is found exit the program"
              n558 = Stop(stop? (T)=w953) -> ()
            }
            frame #2 {
              w964 = 0
              n559 = local read "Select COM port"() -> (w954:refnum<visa-resource-name>)
              n560 = local read "baud rate"() -> (w955:u32)
              n561 = call "VISA Configure Serial Port (Instr)mod.vi"("VISA resource name"=w954, "Enable Termination\nChar (T)"=FALSE, "baud rate (9600)"=w955, "data bits (8)"=8, "parity (0:none)"=w964, "error in (no error)"=w957, "flow control (0:none)"=w964) -> ("VISA resource name out"=w960:refnum<visa-resource-name>, "error out"=w961:errorcluster)  [unwired: 5 in, 2 out]
              n562 = VISA Open(error in (no error)=w961, VISA resource name=w960) -> (VISA resource name=w962:refnum<visa-resource-name>, error out=w963:errorcluster)  [unwired: 3 out]
              n563 = VISA Flush I/O Buffer(VISA resource name=w962, mask (16)=u16 16 ("Maskieren (16)"), error in (no error)=w963) -> (error out=w956:errorcluster)  [unwired: 1 out]
            }
            frame #3 {
              w972 = u16 16  # I/O Receive Buffer mask
              # "Flushes the I/O buffer specified by mask."
              # "Sets the size of the I/O buffer"
              # "Request board ID\nchar. sent \"i\""
              # "Send commend: Request Board ID. CNK will reply with a serial number"
              # "Flushes and discards \ncontents of the \nreceive buffer"
              n564 = local read "Select COM port"() -> (w974:refnum<visa-resource-name>)
              n565 = local read "Input buffer size"() -> (w971:u32)
              n566 = Concatenate Strings("i", "\r") -> (w969:string)
              n567 = VISA Set I/O Buffer Size(VISA resource name=w974, mask (16)=w972, size (4096)=w971, error in (no error)=w967) -> (VISA resource name out=w975:refnum<visa-resource-name>, error out=w973:errorcluster)
              n568 = VISA Flush I/O Buffer(VISA resource name=w975, mask (16)=w972, error in (no error)=w973) -> (VISA resource name out=w977:refnum<visa-resource-name>, error out=w976:errorcluster)
              n569 = VISA Write(VISA resource name=w977, write buffer=w969, error in (no error)=w976) -> (error out=w966:errorcluster)  [unwired: 2 out]
            }
            frame #4 {
              n570 = Wait (ms)(milliseconds to wait=400) -> ()  [unwired: 1 out]
            }
            frame #5 {
              # "If no responce exit application"
              n571 = local read "Select COM port"() -> (w980:refnum<visa-resource-name>)
              n572 = property class="Instr"(reference=w980) -> (reference out=w986:refnum<visa-resource-name>, "Bytes at Port"=w988:u32)  [unwired: 1 in, 1 out]
              n573 = Less Or Equal?(x=w988, y=1) -> (x <= y?=w989:bool)
              n574 = VISA Read(VISA resource name=w986, byte count=w988, error in (no error)=w981) -> (read buffer=w983:string, error out=w982:errorcluster)  [unwired: 2 out]
              n575 = case shown="True" w989 {
                tunnel: w986 -> [_ w994]
                tunnel: w982 -> [_ w993]
                frame False {
                  # "RESET USB = GREEN"
                  n576 = local write "RESET USB"(FALSE) -> ()
                }
                frame True {
                  n577 = stacked-sequence {
                    tunnel: w994 -> [w996 _ _]
                    tunnel: w993 -> [w995 _ _]
                    frame #0 {
                      # "Close VISA"
                      n578 = VISA Close(VISA resource name=w996, error in (no error)=w995) -> ()  [unwired: 1 out]
                    }
                    frame #1 {
                      # "REST USB = RED"
                      n579 = local write "RESET USB"(TRUE) -> ()
                    }
                    frame #2 {
                      n580 = Stop(stop? (T)=TRUE ("Stop? (T)")) -> ()
                    }
                  }
                }
              }
              n581 = Equal?(x=w983, y="") -> (x = y?=w984:bool)
              n582 = case shown="True" w984 {
                tunnel: [w990 "No Responce"] -> w979
                tunnel: w983 -> [w990 _]
                frame False {
                }
                frame True {
                }
              }
              n583 = local write "Message"(w979) -> ()
            }
            frame #6 {
              # "Once program responds with ID it returns to the main() to continue to collect data"
              n584 = Wait (ms)(milliseconds to wait=1000) -> ()  [unwired: 1 out]
            }
          }
        }
        frame #1 {
          n585 = flat-sequence {
            frame #0 {
              n586 = stacked-sequence {
                seq-local: [w1000 _ _ _ _] -> [_ _ _ _ w1041]
                seq-local: [_ _ _ _ w1040] -> [_ _ _ _ _]
                frame #0 {
                  w1012 = u16 16  # I/O Receive Buffer mask
                  # "1. Sets the size of the I/O buffer.\n2.  Flushes the I/O buffer specified by mask."
                  # "Flushes and discards \ncontents of the \nreceive buffer"
                  n587 = local read "Input buffer size"() -> (w1002:u32)
                  n588 = local read "Select COM port"() -> (w1008:refnum<visa-resource-name>)
                  n589 = VISA Set I/O Buffer Size(VISA resource name=w1008, mask (16)=w1012, size (4096)=w1002) -> (VISA resource name out=w1007:refnum<visa-resource-name>, error out=w1001:errorcluster)  [unwired: 1 in]
                  n590 = Concatenate Strings("m", "\r") -> (w1011:string)
                  n591 = local write "RESET USB"(FALSE) -> ()
                  n592 = VISA Flush I/O Buffer(VISA resource name=w1007, mask (16)=w1012, error in (no error)=w1001) -> (VISA resource name out=w1005:refnum<visa-resource-name>, error out=w1006:errorcluster)
                  n593 = VISA Write(VISA resource name=w1005, write buffer=w1011, error in (no error)=w1006) -> (return count=w1003:u32, error out=w1000:errorcluster)  [unwired: 1 out]
                  n594 = local write "# of bytes written"(w1003) -> ()
                }
                frame #1 {
                  n595 = Wait (ms)(milliseconds to wait=100) -> ()  [unwired: 1 out]
                }
                frame #2 {
                  # "1. Determine the length of the string\n2. Maximum number of characters receved by Multimeter + is 7"
                  # "Add remaining nuber of 0s in front"
                  n596 = local read "Select COM port"() -> (w1023:refnum<visa-resource-name>)
                  n597 = String Length(string="Data Rate (u-sec)") -> (length=w1022:i32)
                  n598 = Subtract(x=7, y=w1022) -> (x-y=w1017:i32)
                  n599 = Less?(x=w1017, y=0) -> (x < y?=w1020:bool)
                  n600 = case shown="True" w1020 {
                    tunnel: [w1024 0] -> w1018
                    tunnel: w1017 -> [w1024 _]
                    frame False {
                    }
                    frame True {
                    }
                  }
                  n601 = for {
                    N: w1018 -> [_]
                    tunnel: ["0"] -> w1016 mode=indexing
                  }
                  n602 = Concatenate Strings(w1016, "Data Rate (u-sec)") -> (w1014:string)
                  n603 = VISA Write(VISA resource name=w1023, write buffer=w1014) -> ()  [unwired: 1 in, 3 out]
                }
                frame #3 {
                  n604 = Wait (ms)(milliseconds to wait=50) -> ()  [unwired: 1 out]
                }
                frame #4 {
                  # "Data is collected and sent asyncronously"
                  n605 = local read "Select COM port"() -> (w1028:refnum<visa-resource-name>)
                  n606 = while {
                    tunnel: w1028 -> [w1052]
                    tunnel: w1041 -> [w1055]
                    tunnel: [w1054] -> w1040
                    tunnel: [w1053] -> w1037
                    tunnel: [w1049] -> w1029 mode=concatenating
                    i -> [w1045]
                    stop <- "Stop Data Aquisition" stop-if-true
                    n607 = property class="Instr"(reference=w1052) -> (reference out=w1051:refnum<visa-resource-name>, "Bytes at Port"=w1048:u32)  [unwired: 1 in, 1 out]
                    n608 = Equal?(x=w1045, y=1) -> (x = y?=w1046:bool)
                    n609 = VISA Read(VISA resource name=w1051, byte count=w1048, error in (no error)=w1055) -> (read buffer=w1043:string, return count=w1053:u32, error out=w1054:errorcluster)  [unwired: 1 out]
                    n610 = case shown="True" w1046 {
                      tunnel: w1043 -> [w1056 w1058]
                      tunnel: [w1056 w1057] -> w1042
                      frame False {
                      }
                      frame True {
                        w1059 = 50
                        n611 = String Subset(string=w1058, offset (0)=0, length (rest)=w1059) -> (substring=w1061:string)
                        n612 = local write "Message"(w1061) -> ()
                        n613 = String Subset(string=w1058, offset (0)=w1059) -> (substring=w1057:string)  [unwired: 1 in]
                      }
                    }
                    n614 = local write "Bytes at Port"(w1048) -> ()
                    n615 = Wait (ms)(milliseconds to wait="Loop Delay") -> ()  [unwired: 1 out]
                    n616 = String To Byte Array(string=w1042) -> (unsigned byte array=w1049:u8[])
                  }
                  n617 = local write "Actual bytes read"(w1037) -> ()
                  n618 = call "LA_data_decode_Rev02.vi"("Data In"=w1029) -> ("Data Packs"=→"Number of Data Packs":dbl, "Data Bytes"=→"Data Bytes":dbl, "RG14"=w1033:u8[])  [unwired: 7 in, 1 out]
                  n619 = call "Convert to Dynamic Data8"("Array"=w1033) -> ("Dynamic Data Type"=w1038:dynamicdata)  [unwired: 3 in]
                  n620 = Merge Signals(w1038) -> (→"Data Waveform":dynamicdata)
                  n621 = property on="Data Waveform" class="WFGraph (strict)"("YScale.Maximum"="maximum", "YScale.Minimum"="minimum") -> ()  [unwired: 2 in, 2 out]
                  n622 = property on="Data Waveform" class="WFGraph (strict)"("XScale.Maximum"="X-max", "XScale.Minimum"="X-min") -> ()  [unwired: 2 in, 2 out]
                }
              }
            }
            frame #1 {
              n623 = local read "Select COM port"() -> (w1062:refnum<visa-resource-name>)
              n624 = stacked-sequence {
                tunnel: w1062 -> [_ w1064 _ _ _]
                frame #0 {
                  n625 = Wait (ms)(milliseconds to wait=1000) -> ()  [unwired: 1 out]
                }
                frame #1 {
                  n626 = call "g_send.vi"("Input buffer size"=16384, "USB Interface Name"=w1064) -> ()  [unwired: 9 in, 1 out]
                }
                frame #2 {
                  n627 = Wait (ms)(milliseconds to wait=5) -> ()  [unwired: 1 out]
                }
                frame #3 {
                  n628 = local read "Select COM port"() -> (w1067:refnum<visa-resource-name>)
                  n629 = VISA Close(VISA resource name=w1067) -> ()  [unwired: 1 in, 1 out]
                }
                frame #4 {
                  n630 = Stop(stop? (T)=TRUE ("Stop? (T)")) -> ()
                }
              }
            }
          }
        }
      }
    }
    frame "100 Hz (24 bit)" {
      n631 = stacked-sequence {
        tunnel: [_ "Select path and filename"] -> w1070
        frame #0 {
          n632 = stacked-sequence {
            seq-local: [w1078 _ _ _ _ _ _] -> [_ _ w1086 _ _ _ _]
            seq-local: [_ _ w1085 _ _ _ _] -> [_ _ _ w1098 _ _ _]
            seq-local: [_ _ _ w1097 _ _ _] -> [_ _ _ _ _ w1111 _]
            seq-local: [w1076 _ _ _ _ _ _] -> [_ w1081 _ _ _ _ _]
            frame #0 {
              # "Looking for available com ports"
              n633 = call "No_COM_port_found_EXIT.vi"("Message In"="No COM port found") -> ("STOP"=w1076:bool, "Message Out"=w1080:string, "COM PORTS"=→"Available COM ports":string[], "error out"=w1078:errorcluster)  [unwired: 6 in, 1 out]
              n634 = local write "Message"(w1080) -> ()
            }
            frame #1 {
              # "If no COM port is found exit the program"
              n635 = Stop(stop? (T)=w1081) -> ()
            }
            frame #2 {
              w1095 = 0
              n636 = call "VISA Configure Serial Port (Instr)mod.vi"("VISA resource name"="Select COM port", "Enable Termination\nChar (T)"=FALSE, "baud rate (9600)"="baud rate", "data bits (8)"=8, "parity (0:none)"=w1095, "error in (no error)"=w1086, "flow control (0:none)"=w1095) -> ("VISA resource name out"=w1091:refnum<visa-resource-name>, "Name"=→"Connected to:":string, "Name 2"=→"Connected to Name":string, "error out"=w1092:errorcluster)  [unwired: 5 in]
              n637 = VISA Open(error in (no error)=w1092, VISA resource name=w1091) -> (VISA resource name=w1093:refnum<visa-resource-name>, error out=w1094:errorcluster)  [unwired: 3 out]
              n638 = VISA Flush I/O Buffer(VISA resource name=w1093, mask (16)=u16 16 ("Maskieren (16)"), error in (no error)=w1094) -> (error out=w1085:errorcluster)  [unwired: 1 out]
            }
            frame #3 {
              w1102 = u16 16  # I/O Receive Buffer mask
              # "Request board ID\nchar. sent \"i\""
              # "Send commend: Request Board ID. CNK will reply with a serial number"
              # "Flushes and discards \ncontents of the \nreceive buffer"
              n639 = local read "Select COM port"() -> (w1104:refnum<visa-resource-name>)
              n640 = local read "Input buffer size"() -> (w1101:u32)
              n641 = Concatenate Strings("i", "\r") -> (w1100:string)
              n642 = VISA Set I/O Buffer Size(VISA resource name=w1104, mask (16)=w1102, size (4096)=w1101, error in (no error)=w1098) -> (VISA resource name out=w1105:refnum<visa-resource-name>, error out=w1103:errorcluster)
              n643 = VISA Flush I/O Buffer(VISA resource name=w1105, mask (16)=w1102, error in (no error)=w1103) -> (VISA resource name out=w1107:refnum<visa-resource-name>, error out=w1106:errorcluster)
              n644 = VISA Write(VISA resource name=w1107, write buffer=w1100, error in (no error)=w1106) -> (error out=w1097:errorcluster)  [unwired: 2 out]
            }
            frame #4 {
              n645 = Wait (ms)(milliseconds to wait=400) -> ()  [unwired: 1 out]
            }
            frame #5 {
              # "If no responce exit application"
              n646 = local read "Select COM port"() -> (w1110:refnum<visa-resource-name>)
              n647 = property class="Instr"(reference=w1110) -> (reference out=w1116:refnum<visa-resource-name>, "Bytes at Port"=w1118:u32)  [unwired: 1 in, 1 out]
              n648 = Less Or Equal?(x=w1118, y=1) -> (x <= y?=w1119:bool)
              n649 = VISA Read(VISA resource name=w1116, byte count=w1118, error in (no error)=w1111) -> (read buffer=w1113:string, error out=w1109:errorcluster)  [unwired: 2 out]
              n650 = case shown="True" w1119 {
                tunnel: w1116 -> [_ w1123]
                tunnel: w1109 -> [_ w1124]
                frame False {
                  # "RESET USB = GREEN"
                  n651 = local write "RESET USB"(FALSE) -> ()
                }
                frame True {
                  n652 = stacked-sequence {
                    tunnel: w1123 -> [w1126 _ _]
                    tunnel: w1124 -> [w1125 _ _]
                    frame #0 {
                      # "Close VISA"
                      n653 = VISA Close(VISA resource name=w1126, error in (no error)=w1125) -> ()  [unwired: 1 out]
                    }
                    frame #1 {
                      # "REST USB = RED"
                      n654 = local write "RESET USB"(TRUE) -> ()
                    }
                    frame #2 {
                      n655 = Stop(stop? (T)=TRUE ("Stop? (T)")) -> ()
                    }
                  }
                }
              }
              n656 = Equal?(x=w1113, y="") -> (x = y?=w1114:bool)
              n657 = case shown="True" w1114 {
                tunnel: [w1120 "No Responce"] -> w1112
                tunnel: w1113 -> [w1120 _]
                frame False {
                }
                frame True {
                }
              }
              n658 = local write "Message"(w1112) -> ()
            }
            frame #6 {
              # "Once program responds with ID it returns to the main() to continue to collect data"
              n659 = Wait (ms)(milliseconds to wait=1000) -> ()  [unwired: 1 out]
            }
          }
        }
        frame #1 {
          # "Low frequency o-scope"
          # "Boar ID is received in the frame number 0"
          n660 = while {
            tunnel: "Select path and filename" -> [w1135]
            stop <- TRUE continue-if-true
            n661 = local read "Select COM port"() -> (w1132:refnum<visa-resource-name>)
            n662 = call "Send_control_char_and_STOP.vi"("Select COM port"=w1132, "STOP"="STOP", "Char to send"="Char to send", "Send Char"="Async send character") -> ()  [unwired: 8 in]
            n663 = Or(x="Single shot", y="Continuous") -> (x .or. y?=w1139:bool)
            n664 = case shown="True" w1139 {
              tunnel: w1135 -> [_ w1141]
              frame False {
              }
              frame True {
                n665 = stacked-sequence {
                  seq-local: [_ _ w1164 _ _ _ _ _ _ _ _ _ _] -> [_ _ _ _ w1197 _ _ _ _ _ _ _ _]
                  seq-local: [_ _ _ _ w1207 _ _ _ _ _ _ _ _] -> [_ _ _ _ _ _ _ _ _ _ _ _ _]
                  seq-local: [_ _ _ _ _ _ _ _ "Range select INPUT2" _ _ _ _] -> [_ _ _ _ _ _ _ _ _ w1328 _ _ _]
                  seq-local: [_ _ _ _ _ _ _ _ w1313 _ _ _ _] -> [_ _ _ _ _ _ _ _ _ w1327 _ _ w1376]
                  seq-local: [_ _ _ _ _ _ _ _ _ w1328 _ _ _] -> [_ _ _ _ _ _ _ _ _ _ _ _ _]
                  seq-local: [_ w1151 _ _ _ _ _ _ _ _ _ _ _] -> [_ _ w1163 _ _ _ w1219 _ _ _ _ _ _]
                  seq-local: [_ _ w1165 _ _ _ _ _ _ _ _ _ _] -> [_ _ _ w1183 _ _ _ _ _ _ _ _ _]
                  seq-local: [_ _ _ _ _ _ w1218 _ _ _ _ _ _] -> [_ _ _ _ _ _ _ _ w1266 _ _ _ _]
                  tunnel: w1141 -> [_ _ _ _ _ _ _ _ w1257 _ _ _ _]
                  frame #0 {
                    n666 = flat-sequence {
                      frame #0 {
                        # "CH0"
                        # "Send range multipliers"
                        n667 = local read "Auto / Manual"() -> (w1144:bool)
                        n668 = local read "Range select INPUT1"() -> (w1142:u16)
                        n669 = local read "Select COM port"() -> (w1143:refnum<visa-resource-name>)
                        n670 = call "CH0_Manual_range_select.vi"("Select COM port"=w1143, "EN"=w1144, "IN1 L"=w1142) -> ()  [unwired: 8 in, 1 out]
                      }
                      frame #1 {
                        # "CH1"
                        # "Send Range Multipliers"
                        n671 = local read "Auto / Manual"() -> (w1147:bool)
                        n672 = local read "Range select INPUT2"() -> (w1146:u16)
                        n673 = local read "Select COM port"() -> (w1145:refnum<visa-resource-name>)
                        n674 = call "CH1_Manual_range_select.vi"("CH1"=w1146, "EN"=w1147, "Select COM port"=w1145) -> ()  [unwired: 8 in, 1 out]
                      }
                    }
                  }
                  frame #1 {
                    w1162 = u16 16  # I/O Receive Buffer mask
                    # "This case is required for both manual and autorange. D request calibrated dividers and shift values from memory"
                    # "Flushes and discards \ncontents of the \nreceive buffer"
                    # "Once the boar ID is received send the next command.\n\"D\" places a request to send back dividors and all the \ncalibration values"
                    n675 = local read "Select COM port"() -> (w1155:refnum<visa-resource-name>)
                    n676 = Concatenate Strings("D", "\r") -> (w1161:string)
                    n677 = Not(x="Auto / Manual") -> (.not. x?=w1150:bool)
                    n678 = VISA Set I/O Buffer Size(VISA resource name=w1155, mask (16)=w1162, size (4096)="Input buffer size") -> (VISA resource name out=w1154:refnum<visa-resource-name>, error out=w1156:errorcluster)  [unwired: 1 in]
                    n679 = property on="Auto / Manual" class="Bool (strict)"("Blinking"=w1150) -> ()  [unwired: 2 in, 2 out]
                    n680 = VISA Flush I/O Buffer(VISA resource name=w1154, mask (16)=w1162, error in (no error)=w1156) -> (VISA resource name out=w1152:refnum<visa-resource-name>, error out=w1153:errorcluster)
                    n681 = VISA Write(VISA resource name=w1152, write buffer=w1161, error in (no error)=w1153) -> (return count=→"# of bytes written":u32, error out=w1151:errorcluster)  [unwired: 1 out]
                    n682 = local write "RESET USB"(FALSE) -> ()
                  }
                  frame #2 {
                    # "Byte 0          : divider CH0 is on the right so it is Input 2 on the right\nByte 1          : divider CH1 is on the left so it is Input 1 on the left\nByte 2,3,4,5 : Shift voltage CH0. byte[2] is LSB byte[5] is MSB\nByte 7,8,9,10: Shift voltage CH0. byte[7] is LSB byte[10] is MSB"
                    n683 = flat-sequence {
                      tunnel: [w1169] -> w1165
                      tunnel: [w1168] -> w1164
                      tunnel: w1163 -> [w1167]
                      frame #0 {
                        n684 = Wait (ms)(milliseconds to wait=2) -> ()  [unwired: 1 out]
                      }
                      frame #1 {
                        n685 = while {
                          tunnel: [w1173] -> w1169
                          tunnel: [w1172] -> w1168
                          tunnel: w1167 -> [w1171]
                          stop <- w1178 stop-if-true
                          # "Responce to 'D' request"
                          # "10 bytes"
                          n686 = local read "Select COM port"() -> (w1176:refnum<visa-resource-name>)
                          n687 = property class="Instr"(reference=w1176, error in=w1171) -> (reference out=w1174:refnum<visa-resource-name>, error out=w1175:errorcluster, "Bytes at Port"=w1170:u32)
                          n688 = local write "Bytes at Port"(w1170) -> ()
                          n689 = VISA Read(VISA resource name=w1174, byte count=w1170, error in (no error)=w1175) -> (read buffer=w1173:string, error out=w1172:errorcluster)  [unwired: 2 out]
                          n690 = Greater?(x=w1170, y=9) -> (0:w1178:bool)
                        }
                      }
                    }
                  }
                  frame #3 {
                    w1187 = 0
                    # "Shift INPUT 1L works"
                    # "Byte 2,3,4,5: Shift voltage CH0"
                    # "This function decodes multiplier and shift values sent from CNK Handheld"
                    # "Converts received dividers and \nshifters into decimal values"
                    # "Read back channel multipliers\nand level shifters."
                    n691 = String To Byte Array(string=w1183) -> (unsigned byte array=w1184:u8[])
                    "Array" <- w1184
                    n692 = call "divider_and_offset_Rev_03.vi"("Char Array In"=w1184, "Control Char"="D") -> ("Div In2 Rgt Ind"=→"Range Sel IN2 in":dbl, "Div In1 Lft Ind"=→"Range Sel IN1 in":dbl, "Div In1 Lft"=w1190:dbl, "Div In2 Rgt"=w1182:dbl, "INPUT2 shift sign"=→"INPUT2 shift sign":dbl, "INPUT1 shift sign"=→"INPU1 shift sign":dbl, "Shift IN2 R ch1"=w1189:dbl, "Shift IN1 L ch0"=w1181:dbl)  [unwired: 5 in, 1 out]
                    n693 = local write "Divider INPUT1 L"(w1190) -> ()
                    n694 = local write "Divider INPUT2 R"(w1182) -> ()
                    n695 = Select(t=w1181, s="SHIFT INPUT1 L SEL", f=w1187) -> (s? t:f=→"Shift INPUT1 L":dbl)
                    n696 = Select(t=w1189, s="SHIFT INPUT2 R SEL", f=w1187) -> (s? t:f=→"Shift INPUT2 R":dbl)
                    "String" <- w1183
                  }
                  frame #4 {
                    w1201 = u16 16  # I/O Receive Buffer mask
                    # "H - high speed"
                    # "Get the first character.\nSecond character is <CR>"
                    # "MAIN COMMAND"
                    n697 = call "CommandSelect.vi"("Config Sel"="Send New Configuration", "A/D Settings"="A/D settings", "Command"="Command") -> ("Command Out"=w1195:string)  [unwired: 8 in]
                    n698 = local read "Select COM port"() -> (w1200:refnum<visa-resource-name>)
                    n699 = VISA Flush I/O Buffer(VISA resource name=w1200, mask (16)=w1201, error in (no error)=w1197) -> (VISA resource name out=w1204:refnum<visa-resource-name>, error out=w1203:errorcluster)
                    n700 = Concatenate Strings(w1195, "\r") -> (w1205:string)
                    n701 = VISA Write(VISA resource name=w1204, write buffer=w1205, error in (no error)=w1203) -> (error out=w1207:errorcluster)  [unwired: 2 out]
                    n702 = String Subset(string=w1205, length (rest)=1) -> (substring=→"Sent Command":string)  [unwired: 1 in]
                  }
                  frame #5 {
                    # "If received char is not 's' \nthere will be wait period\nof 2 sec"
                    # "Allows enough\ntime for the A/D converter\nto collect the required\n# of samples."
                    n703 = local read "Sent Command"() -> (w1209:string)
                    n704 = case shown="\"H\"" w1209 {
                      tunnel: [u32 0 ("Wait ms") u32 0 ("Wait ms") u32 0 ("Wait ms") u32 0 ("Wait ms") u32 0 ("Wait ms") u32 0 ("Wait ms")] -> w1211
                      frame "O", Default {
                        # "Plot the chart case 40"
                      }
                      frame "H" {
                      }
                      frame "s" {
                        # "256 samples"
                      }
                      frame "N" {
                      }
                      frame "0" {
                      }
                      frame "S" {
                        # "2048 samples"
                      }
                    }
                    n705 = Wait (ms)(milliseconds to wait=w1211) -> (millisecond timer value=→"Delay":u32)
                  }
                  frame #6 {
                    # "Wait here untill all the data is received"
                    n706 = while {
                      tunnel: [w1232] -> w1218
                      tunnel: w1219 -> [w1220]
                      i -> [w1222]
                      stop <- w1224 stop-if-true
                      n707 = local read "Select COM port"() -> (w1227:refnum<visa-resource-name>)
                      n708 = property class="Instr"(reference=w1227, error in=w1220) -> (error out=w1232:errorcluster, "Bytes at Port"=w1229:u32)  [unwired: 1 out]
                      n709 = Divide(x=w1229, y=3) -> (x/y=→"Number of data points":dbl)
                      n710 = local write "Bytes at Port"(w1229) -> ()
                      n711 = local read "Sent Command"() -> (w1226:string)
                      n712 = case shown="\"S\"" w1226 {
                        tunnel: [1529 0 0 0 12287 12287 12287] -> w1231
                        frame "s" {
                        }
                        frame "H" {
                        }
                        frame Default {
                        }
                        frame "W" {
                        }
                        frame "N" {
                        }
                        frame "O" {
                        }
                        frame "S" {
                          # "Number of bytes"
                        }
                      }
                      n713 = Greater?(x=w1229, y=w1231) -> (0:w1225:bool)
                      n714 = Greater?(x=w1222, y=1000000) -> (0:w1223:bool)
                      n715 = Or(x=w1223, y=w1225) -> (x .or. y?=w1224:bool)
                      "Loop Count" <- w1222
                    }
                  }
                  frame #7 {
                    # "lowest 10 ms"
                    n716 = local read "Sent Command"() -> (w1241:string)
                    n717 = case shown="\"False\", Default" w1241 {
                      frame "False", Default {
                      }
                      frame "H" {
                        n718 = stacked-sequence {
                          frame #0 {
                            n719 = local read "Select COM port"() -> (w1244:refnum<visa-resource-name>)
                            n720 = property class="Instr"(reference=w1244) -> (reference out=w1245:refnum<visa-resource-name>, "Bytes at Port"=w1243:u32)  [unwired: 1 in, 1 out]
                            n721 = VISA Read(VISA resource name=w1245, byte count=w1243) -> (read buffer=w1242:string)  [unwired: 1 in, 3 out]
                            n722 = local write "Message"(w1242) -> ()
                          }
                          frame #1 {
                            n723 = Wait (ms)(milliseconds to wait=u32 50 ("Wait ms")) -> ()  [unwired: 1 out]
                          }
                          frame #2 {
                            n724 = disable-structure shown="Disabled" {
                              frame Disabled {
                                w1252 = u16 16  # I/O Receive Buffer mask
                                n725 = local read "Select COM port"() -> (w1254:refnum<visa-resource-name>)
                                n726 = VISA Flush I/O Buffer(VISA resource name=w1254, mask (16)=w1252) -> (VISA resource name out=w1253:refnum<visa-resource-name>, error out=w1250:errorcluster)  [unwired: 1 in]
                                n727 = Concatenate Strings("S", "\r") -> (w1249:string)
                                n728 = VISA Write(VISA resource name=w1253, write buffer=w1249, error in (no error)=w1250) -> ()  [unwired: 3 out]
                                n729 = String Subset(string=w1249, length (rest)=1) -> (substring=w1247:string)  [unwired: 1 in]
                                n730 = local write "Sent Command"(w1247) -> ()
                              }
                              frame Enabled {
                              }
                            }
                          }
                          frame #3 {
                            n731 = disable-structure shown="Disabled" {
                              frame Disabled {
                                n732 = Wait (ms)(milliseconds to wait=u32 1500 ("Wait ms")) -> ()  [unwired: 1 out]
                              }
                              frame Enabled {
                              }
                            }
                          }
                        }
                      }
                    }
                    n733 = Wait (ms)(milliseconds to wait="Refresh Delay") -> ()  [unwired: 1 out]
                  }
                  frame #8 {
                    # "FFT"
                    # "AD data"
                    n734 = local read "Sent Command"() -> (w1263:string)
                    n735 = local read "Select COM port"() -> (w1279:refnum<visa-resource-name>)
                    n736 = property class="Instr"(reference=w1279, error in=w1266) -> (reference out=w1323:refnum<visa-resource-name>, error out=w1321:errorcluster, "Bytes at Port"=w1322:u32)
                    "Bytes at Port" <- w1322
                    n737 = local read "VDC INPUT2"() -> (w1292:dbl)
                    n738 = call "Exit_prog.vi"("EN/DIS"=TRUE, "error in (no error)"=w1321, "InputStr"=w1263, "Bytes to read"=w1322, "USB Interface Name"=w1279) -> ("error out"=w1320:errorcluster, "RESET USB"=→"RESET USB":bool)  [unwired: 4 in, 1 out]
                    n739 = property on="FFT" class="WFGraph (strict)"("XScale.Maximum"="Zoom In Graph ---> 2") -> ()  [unwired: 2 in, 2 out]
                    n740 = property on="Waveform Graph 2" class="WFGraph (strict)"("XScale.Maximum"="Zoom In Graph --->") -> ()  [unwired: 2 in, 2 out]
                    n741 = property on="Voltage" class="WFGraph (strict)"("XScale.Maximum"="Zoom In Graph --->") -> ()  [unwired: 2 in, 2 out]
                    n742 = property on="Voltage" class="WFGraph (strict)"("XScale.Minimum"=0.0) -> ()  [unwired: 2 in, 2 out]
                    n743 = VISA Read(VISA resource name=w1323, byte count=w1322, error in (no error)=w1320) -> (read buffer=w1272:string, return count=w1293:u32, error out=w1294:errorcluster)  [unwired: 1 out]
                    "Actual bytes read" <- w1293
                    n744 = call "Store_Val2_CH2.vi"("Store"="Store Value 2 IN2", "Vin"=w1292) -> ("Saved Value"=→"Saved Value 2 IN2":dbl)  [unwired: 9 in]
                    n745 = Divide(x=w1293, y=3) -> (x/y=→"Number of Samples":dbl)
                    n746 = String To Byte Array(string=w1272) -> (unsigned byte array=w1305:u8[])
                    n747 = local read "Shift INPUT2 R"() -> (w1296:dbl)
                    n748 = property on="DC Filter" class="Bool (strict)"("Blinking"="DC Filter") -> ()  [unwired: 2 in, 2 out]
                    n749 = local read "Divider INPUT1 L"() -> (w1258:dbl)
                    n750 = local read "Divider INPUT2 R"() -> (w1259:dbl)
                    n751 = local read "Shift INPUT1 L"() -> (w1268:dbl)
                    n752 = call "compute_engine_CH0CH1_Rev01.vi"("INPUT 1L Loc"="INPUT 1L Loc", "INPUT 2R Loc"="INPUT 2R Loc", "Array In"=w1305, "Input Select"="View", "Control Character"=w1263, "Divider INPUT1L"=w1258, "Number of datapoints"=w1293, "Divider INPUT2R"=w1259, "DC Filter"="DC Filter", "Shift INPUT 1L"=w1268, "AC/DC INPUT2"="AC/DC INPUT 1", "Shift INPUT 2R"=w1296, "AC /DC INPUT1"="AC /DC INPUT 2") -> ("INPUT2"=w1273:dbl[], "VRMS INPUT1"=→"VRMS INPUT1":dbl, "INPUT1"=w1262:dbl[], "VDC INPUT2"=→"VDC INPUT2":dbl, "VRMS INPUT2"=→"VRMS INPUT2":dbl, "VDC INPUT1"=→"VDC INPUT1":dbl)  [unwired: 5 in, 4 out]
                    n753 = local read "VDC INPUT1"() -> (w1285:dbl)
                    n754 = local read "VDC INPUT2"() -> (w1282:dbl)
                    n755 = local read "Select COM port"() -> (w1295:refnum<visa-resource-name>)
                    n756 = local read "A/D settings"() -> (w1290:u16)
                    n757 = case shown="0, Default" w1290 {
                      tunnel: [0.00028054795 ("dt") 1.75439e-05] -> w1261
                      frame 1 {
                        # "Set dt"
                      }
                      frame 0, Default {
                        # "Dt for 57 ksps"
                        # "Set dt"
                      }
                    }
                    n758 = call "FFTvi.vi"("Time Delta"=w1261, "Voltage INPUT2"=w1273, "Voltage INPUT1"=w1262) -> ("FFT"=→"FFT":dynamicdata)  [unwired: 8 in]
                    n759 = call "Input selector.vi"("dt"=w1261, "Voltage INPUT2"=w1273, "Voltage INPUT1"=w1262, "Ring"="View") -> ("INPUT2 (Hz)"=→"INPUT1 VAC Hz":dbl, "INPUT1 (Hz)"=→"INPUT2 VAC Hz":dbl, "Sig Out"=w1276:dynamicdata)  [unwired: 2 in, 3 out]
                    "Voltage" <- w1276
                    "Waveform Graph 2" <- w1276
                    n760 = call "Data Store.vi"("Store Value CH0"="Store Value 1 IN2", "VDC INPUT2"=w1282, "VDC INPUT1"=w1285, "Store Value 2 IN1"="Store Value 2 IN1", "Store Value 1 IN1"="Store Value 1 IN1") -> ("Saved Value 2 IN1"=→"Saved Value 2 IN1":dbl, "Saved Value 1 IN1"=→"Saved Value 1 IN1":dbl, "Saved Value CH0"=→"Saved Value 1 IN2":dbl)  [unwired: 4 in]
                    n761 = VISA Flush I/O Buffer(VISA resource name=w1295, mask (16)=16, error in (no error)=w1294) -> (error out=w1313:errorcluster)  [unwired: 1 out]
                    n762 = call "Overload.vi"("INPUT2 Range"="Range select INPUT2", "INPUT1 Range"="Range select INPUT1", "CH1"=w1262, "INPUT 1"=w1273) -> ("CH1 MIN"=→"VMIN CH1":dbl, "CH0 MIN"=→"VMIN IN1":dbl, "CH0 MAX"=w1316:dbl, "OL INPUT1"=w1307:bool, "CH1 MAX"=w1315:dbl, "OL CH1"=w1310:bool)  [unwired: 2 in]
                    "OL IN2" <- w1310
                    "OL IN1" <- w1307
                    "VMAX IN1" <- w1316
                    "VMAX CH1" <- w1315
                    n763 = Subtract(x=w1316, y=w1315) -> (x-y=→"IN1 - IN2 V shift":dbl)
                    n764 = Divide(x=w1316, y=w1315) -> (x/y=→"IN1/IN2 V gain":dbl)
                    n765 = call "Record Data.vi"("Voltage"=w1276, "Continuous Rec Data CH0"="Continuous Rec Data CH0", "Record single value"="Record single value", "Select path and filename"=w1257) -> ()  [unwired: 8 in]
                    n766 = property on="OL IN1" class="Bool (strict)"("Blinking"=w1307) -> ()  [unwired: 2 in, 2 out]
                    n767 = call "CH1_Address_decoder_calibration.vi"("Range IN"="Range select INPUT2") -> ()  [unwired: 7 in, 4 out]
                    n768 = property on="OL IN2" class="Bool (strict)"("Blinking"=w1310) -> ()  [unwired: 2 in, 2 out]
                  }
                  frame #9 {
                    # "Calibration block"
                    n769 = case shown="True" "Enable cal" {
                      tunnel: w1327 -> [_ w1358]
                      frame False {
                      }
                      frame True {
                        # "00000008\n00000009\n00000010\n00000011\n00000041\n\n00000016\n00000017\n00000018\n00000019\n00000043\n\n00000024\n00000025\n00000026\n00000027\n00000045\n\n00000032\n00000033\n00000034\n00000035\n00000047"
                        # "INPUT 2 RIGHT"
                        # "INPUT 1 LEFT"
                        n770 = local read "Select COM port"() -> (w1331:refnum<visa-resource-name>)
                        n771 = local read "Range select INPUT2"() -> (w1332:u16)
                        n772 = local read "Saved Value 1 IN2"() -> (w1341:dbl)
                        n773 = call "Shift_Value_CH1_calibration_Rev02x.vi"("Saved Val IN2"=w1341, "Enable memory wright"="Enable memory wright", "INPUT2 R range in"=w1332, "USB Interface Name"=w1331, "Cal Voltage IN2"="Cal Voltage IN2", "WRITE"="WRITE INPUT2", "Sign Value"="Value of sign CH1") -> ("MB address"=→"MB address 2":string, "MB value"=→"MB  data 2":u8, "Cal to Saved IN2"=→"Cal to Saved IN2":dbl, "UB address"=→"UB address 2":string, "HB address"=→"HB address 2":string, "LB address"=→"LB address 2":string, "UB value"=→"UB data 2":u8, "Reply 1"=→"Reply 5":string, "Reply 4"=→"Reply 8":string, "CH1 shift value uV"=→"CH1 Shift value uV":dbl, "CH1shift val HEX uV"=→"CH1 shift val HEX uV":u32, "Reply 2"=→"Reply 6":string, "Sign Addrss"=→"Sign Address 2":string, "HB value"=→"HB data 2":u8, "LB value"=→"LB data 2":u8, "Reply 3"=→"Reply 7":string)  [unwired: 4 in, 1 out]
                        n774 = local read "Select COM port"() -> (w1371:refnum<visa-resource-name>)
                        n775 = local read "Range select INPUT1"() -> (w1370:u16)
                        n776 = local read "Saved Value 1 IN1"() -> (w1342:dbl)
                        n777 = call "Shift_Value_CH0_calibration_Rev03x.vi"("IN1 Shift Val1"=w1342, "Enable memory wright"="Enable memory wright", "Range IN1"=w1370, "USB Interface Name"=w1371, "error in (no error)"=w1358, "WRITE"="WRITE INPUT1", "Sign Value"="Value of sign") -> ("MB address"=→"MB address":string, "MB value"=→"MB data":u8, "Reply 1"=→"Reply 1":string, "UB address"=→"UB address":string, "HB address"=→"HB address":string, "LB address"=→"LB address":string, "UB value"=→"UB data":u8, "Reply 2"=→"Reply 2":string, "Data string CH0"=→"Data String CH0":string, "IN1 shift uV"=→"CH0 Shift value uV":dbl, "IN1 shift  HEX uV"=→"CH0 shift val HEX uV":u32, "Reply 3"=→"Reply 3":string, "Sign Addrss"=→"Sign Address":string, "HB value"=→"HB data":u8, "LB value"=→"LB data":u8, "Reply 4"=→"Reply 4":string)  [unwired: 4 in, 1 out]
                      }
                    }
                  }
                  frame #10 {
                    n778 = Wait (ms)(milliseconds to wait=250) -> ()  [unwired: 1 out]
                  }
                  frame #11 {
                    n779 = while {
                      stop <- "PAUSE F1" continue-if-true
                    }
                  }
                  frame #12 {
                    n780 = call <vilib>:"Simple Error Handler.vi"("error in (no error)"=w1376) -> ()  [unwired: 1 in, 8 out]
                  }
                }
              }
            }
            n781 = Wait (ms)(milliseconds to wait=u32 10 ("Zu wartende ms")) -> ()  [unwired: 1 out]
          }
        }
      }
      n782 = case shown="True" "Play Button" {
        tunnel: w1070 -> [_ w1073]
        frame False {
        }
        frame True {
          n783 = call "Play_Rec_Data.vi"("Zoom In Graph --->"="Zoom In Graph ---> 3", "Play Speed"="Play Speed", "Stop Button"="Stop Playing", "Select path and filename"=w1073) -> ("Recorded data"=→"Recorded data":waveform(dbl)[])  [unwired: 7 in]
        }
      }
    }
  }
